vi "Configuration.vi"(10 "Open from\nscan VI":bool, 11 "Measurements":T1(tab)) -> (3 "configured?":bool)   [LabVIEW 2013]
uses:
  InstrControl/Switching/Switching.lvclass
  InstrControl/InstrumentSetup.vi
  general_VIs/globals/QC_MeasurementSetup.vi
  general_VIs/globals/QC_RunInformation.vi
  InstrControl/InstrControl.lvclass
panel:
  in  "Defaults Multimeter":bool
  in  "Multimeter":enum32{"Keithley 2000"}(tab)
  in  "Range Value\n(0.1 - 100)":dbl=100.0 format="%#.2g"
  in  "Range":u16(ring) items=["Auto", "Manual"]
  in  "Function":u16(ring)=3 items=["AC Current", "DC Current", "AC Voltage", "DC Voltage", "2W-Resistance", "4W-Resistance", "Period", "Frequency", "Temperature", "Diode", "Continuity"]
  in  "GPIB Address KE2000":i32=19
  in  "Apply":bool
  in  "Defaults LCR":bool
  in  "LCRs":enum32{"WayneKerr 6440B", "WayneKerr 6425"}(tab)
  in  "AC frequency [Hz]":i32=1000 format="%#.3p"
  in  "RC Configuration":u16(ring) items=["serial", "parallel"]
  in  "AC amplitude [V]":sgl=0.1
  in  "GPIB Address WK6440B":i32=23
  in  "GPIB Address WK6425":i32=17
  in  "AC amplitude [V] WK6425":sgl=0.1 caption="AC amplitude [V]"
  in  "RC Configuration WK6425":u16(ring) caption="RC Configuration" items=["serial", "parallel"]
  in  "AC frequency [Hz] WK6425":i32=1000 caption="AC frequency [Hz]" format="%#.3p"
  in  "VISA address":refnum<visa-resource-name>="COM24" caption="Arduino address"
  out "Programm uploaded?":string="Make sure programme is uploaded to Arduino Uno ->"
  in  "Blank Button":bool
  in  "Matrix address":i32=1
  in  "GPIB address":i32=10
  in  "Mux1 address":i32=4
  in  "Mux2 address":i32=5
  in  "Search Button":bool
  out "DIAGNOSTIC? Response":string
  out "Display Matrix":bool[][](array[boolean])
  in  "No Matrix":bool
  out "X Mapping":string[](array[string])
  out "Y Mapping":string[](array[string])
  in  "Change Preset Parameters":bool
  in  "V_breakdown Limit [V]":dbl=-500.0
  in  "IV Temperature Readout":enum16{"Read Arduino", "Enter manually"}(ring) caption="Temperature Readout"
  in  "IV Ramp down Interval [s]":i32=1 caption="Ramp down Interval [s]"
  in  "IV Ramp down steps [V]":dbl=50.0 caption="Ramp down steps [V]"
  in  "IV Step Interval [s]":i32=10 caption="Step Interval [s]"
  in  "IV Step Size [V]":dbl=10.0 caption="Step Size [V]" format="%.1f"
  in  "IV Final Voltage [V]":dbl=-700.0 caption="Final Voltage [V]" format="%.1f"
  in  "IV Initial Voltage [V]":dbl caption="Initial Voltage [V]" format="%.1f"
  in  "IV Voltage Supply":string(combo)="Keithley 2410"
  in  "Save IV defaults":bool
  in  "V_depletion Limit [V]":dbl=-300.0
  in  "CV LCR Meter":string(combo)="WayneKerr 6440B"
  in  "CV Temperature Readout":enum16{"Read Arduino", "Enter manually"}(ring) caption="Temperature Readout"
  in  "Save CV defaults":bool
  in  "CV Voltage Supply":string(combo)="Keithley 2410"
  in  "CV Initial Voltage [V]":dbl caption="Initial Voltage [V]" format="%.1f"
  in  "CV Final Voltage [V]":dbl=-700.0 caption="Final Voltage [V]" format="%.1f"
  in  "CV Step Size [V]":dbl=10.0 caption="Step Size [V]" format="%.1f"
  in  "CV Step Interval [s]":i32=5 caption="Step Interval [s]"
  in  "CV Ramp down steps [V]":dbl=10.0 caption="Ramp down steps [V]"
  in  "CV Ramp down Interval [s]":i32=1 caption="Ramp down Interval [s]"
  in  "Maximum current fluctuation [%]":dbl=2.0
  in  "Save Stability defaults":bool
  in  "Stability Voltage Supply":string(combo)="Keithley 487"
  in  "Fraction of good strips [%]":dbl=98.0
  in  "Bias Supply":string(combo)="Keithley 487"
  in  "SMU":string(combo)="Keithley 2410"
  in  "C_is Limit [pF/cm]":dbl=1.0
  in  "Save Cis defaults":bool
  in  "Cis Voltage Supply":string(combo)="Keithley 2410"
  in  "Cis Temperature Readout":enum16{"Read Arduino", "Enter manually"}(ring) caption="Temperature Readout"
  in  "Cis LCR Meter":string(combo)="WayneKerr 6440B"
  in  "Cis Ramp down Interval [s]":i32=1 caption="Ramp down Interval [s]"
  in  "Cis Ramp down steps [V]":dbl=50.0 caption="Ramp down steps [V]"
  in  "Cis Step Interval [s]":i32=10 caption="Step Interval [s]"
  in  "Cis Step Size [V]":dbl=10.0 caption="Step Size [V]" format="%.1f"
  in  "Cis Final Voltage [V]":dbl=-700.0 caption="Final Voltage [V]" format="%.1f"
  in  "Cis Initial Voltage [V]":dbl caption="Initial Voltage [V]" format="%.1f"
  in  "Ris Voltmeter":string(combo)="Keithley 2000"
  in  "Ris SMU":string(combo)="Keithley 6517"
  in  "Ris Bias Supply":string(combo)="Keithley 487"
  in  "Ris Temperature Readout":enum16{"Read Arduino", "Enter manually"}(ring) caption="Temperature Readout"
  in  "Save Ris defaults":bool
  in  "Ris Initial Voltage [V]":dbl caption="Initial Voltage [V]" format="%.1f"
  in  "Ris Final Voltage [V]":dbl=-700.0 caption="Final Voltage [V]" format="%.1f"
  in  "Ris Step Size [V]":dbl=10.0 caption="Step Size [V]" format="%.1f"
  in  "Ris Step Interval [s]":i32=10 caption="Step Interval [s]"
  in  "Ris Ramp down steps [V]":dbl=50.0 caption="Ramp down steps [V]"
  in  "Ris Ramp down Interval [s]":i32=1 caption="Ramp down Interval [s]"
  in  "R_is Limit [MOhm]":dbl=100.0
  in  "Supplies":T2(tab)
  in  "Current Limit [µA]":sgl=100.0
  in  "GPIB Address KE2410":i32=24
  in  "GPIB Address KE487":i32=22
  in  "Compliance":u16(ring) items=["20µA", "2mA"]
  in  "Range:":u16(ring) items=["Autorange", "2nA", "20nA", "200nA", "2 microAmp", "20 microAmp", "200 microAmp", "2 milliAmp"]
  in  "Current Limit":u16(ring)=1 items=["OFF", "ON"]
  in  "GPIB Address KE6517":i32=27
  in  "current compliance \nlevel [mA]":dbl=0.0001 format="%.4f"
  in  "compliance/\nmeasurement range (auto:0)":u16(ring)=6 items=["auto / auto", "1 nA / 1.1 V", "10 nA / 11 V", "100 nA / 110 V", "0.001 mA / 110 V", "0.01 mA / 110 V", "0.1 mA / 110 V", "1 mA / 110 V", "10 mA / 110 V", "100 mA / 110 V"]
  in  "GPIB Address KE236":i32=16
  in  "Defaults Supply":bool
  in  "OK Button":bool
  out "X Mapping CB Standard":string[](array[string])
  # "Measurement Configuration"
  # "MUX / Matrix Setup"
  # "Does not apply\nto striptest"
  # "Arduino Configuration"
  # "Multimeter Configuration"
  # "Supply Configuration"
  # "LCR Configuration"
  # "Only for\ninitialisation"
  # "Only for\ninitialisation"
  # "Does not do \nanything yet!"
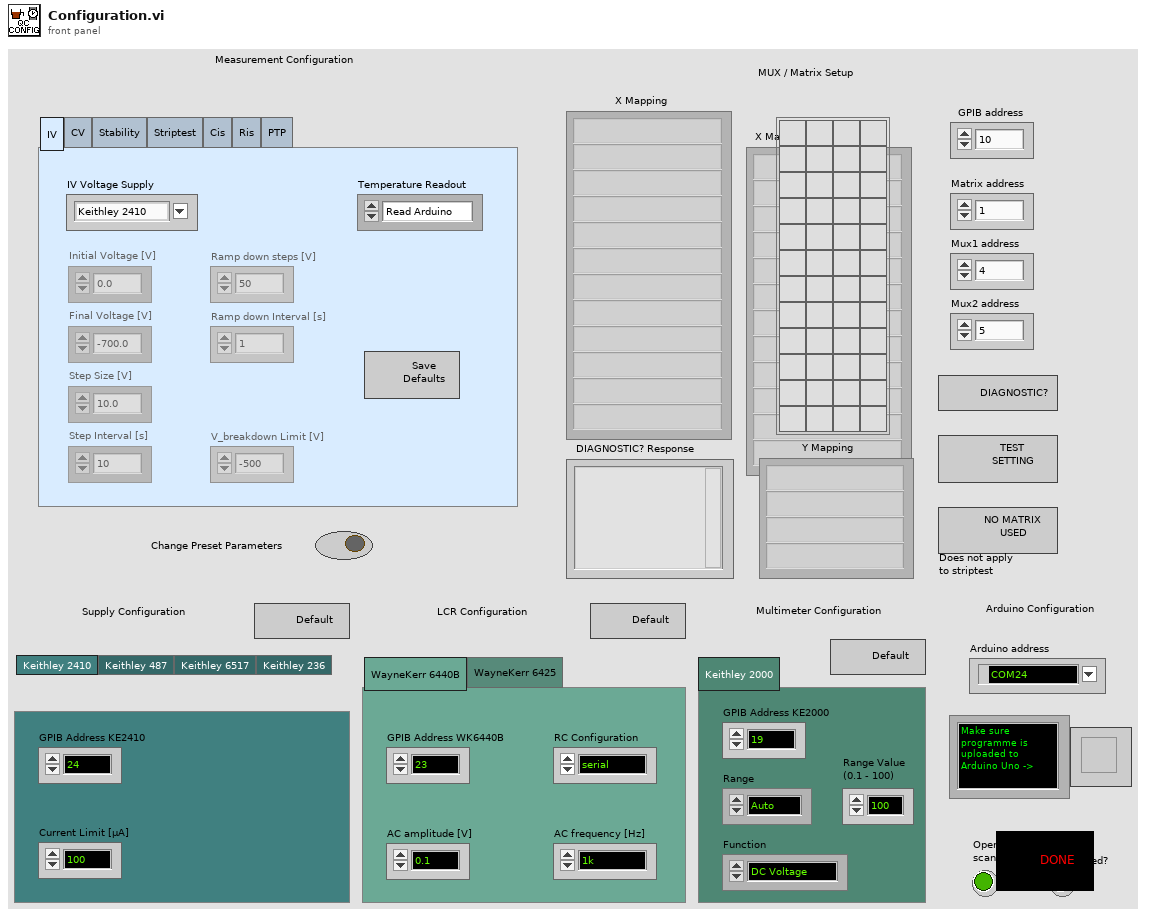
[diagram p1: front panel]
types:
  T1 = enum32{"IV", "CV", "Stability", "Striptest", "Cis", "Ris", "PTP"}
  T2 = enum32{"Keithley 2410", "Keithley 487", "Keithley 6517", "Keithley 236"}
  T3 = enum16{"Reset", "Ground", "Striptest SMU", "Striptest LCR", "IV", "CV", "Interstrip Cap", "Interstrip Res"}
  T4 = cluster{"GPIB address":string, "Matrix address":string, "Mux1 address":string, "Mux2 address":string, "Matrix used?":bool, "Switching":refnum<class "Switching.lvclass">, "Matrix X Channels":cluster{"Bias Supply / SMU LO":i32, "Bias Supply / SMU HI":i32, "CV Box LO":i32, "CV Box HI":i32, "CV Box LO IN":i32, "CV Box HI IN":i32, "Volt meter LO":i32, "Volt meter HI":i32, "Mux1 C1":i32, "Mux1 C2":i32, "Mux2 C1":i32, "Mux2 C2":i32}}
  T5 = cluster{"Supply":refnum<class "SupplyControl.lvclass">, "LCR":refnum<class "LCRControl.lvclass">, "Initial Voltage [V]":dbl, "Final Voltage [V]":dbl, "Step Size [V]":dbl, "Step Interval [s]":i32, "Number Of Steps":u32, "AC frequency [Hz]":i32, "RC Configuration":u16, "AC amplitude [V]":dbl, "Ramp down steps [V]":dbl, "Ramp down Interval [s]":i32, "Set Current Limit?":bool, "Current Limit [µA]":dbl, "Temperature Readout":enum16{"Read Arduino", "Enter manually"}, "Arduino":refnum<class "ArduinoControl.lvclass">, "Supply Name":string, "LCR Name":string, "C_is Limit [pF/cm]":dbl}
  T6 = cluster{"Supply":refnum<class "SupplyControl.lvclass">, "LCR":refnum<class "LCRControl.lvclass">, "Initial Voltage [V]":dbl, "Final Voltage [V]":dbl, "Step Size [V]":dbl, "Step Interval [s]":i32, "Number Of Steps":u32, "AC frequency [Hz]":i32, "RC Configuration":u16, "AC amplitude [V]":dbl, "Ramp down steps [V]":dbl, "Ramp down Interval [s]":i32, "Set Current Limit?":bool, "Current Limit [µA]":dbl, "Temperature Readout":enum16{"Read Arduino", "Enter manually"}, "Arduino":refnum<class "ArduinoControl.lvclass">, "Supply Name":string, "LCR Name":string, "V_depletion Limit [V]":dbl}
  T7 = cluster{"Bias Supply":refnum<class "SupplyControl.lvclass">, "SMU":refnum<class "SupplyControl.lvclass">, "Multimeter":refnum<class "MultimeterControl.lvclass">, "Initial Voltage [V]":dbl, "Final Voltage [V]":dbl, "Step Size [V]":dbl, "Step Interval [s]":i32, "Number Of Steps":u32, "Ramp down steps [V]":dbl, "Ramp down Interval [s]":i32, "Set Current Limit?":bool, "Current Limit [µA]":dbl, "Temperature Readout":enum16{"Read Arduino", "Enter manually"}, "Arduino":refnum<class "ArduinoControl.lvclass">, "Supply Name":string, "SMU Name":string, "Voltmeter Name":string, "R_is Limit [MOhm]":dbl}
  T8 = cluster{"Supply":refnum<class "SupplyControl.lvclass">, "Initial Voltage [V]":dbl, "Final Voltage [V]":dbl, "Step Size [V]":dbl, "Step Interval [s]":i32, "Number Of Steps":u32, "Ramp down steps [V]":dbl, "Ramp down Interval [s]":i32, "Set Current Limit?":bool, "Current Limit [µA]":dbl, "Temperature Readout":enum16{"Read Arduino", "Enter manually"}, "Arduino":refnum<class "ArduinoControl.lvclass">, "Supply Name":string, "V_breakdown Limit [V]":dbl}
  T9 = cluster{"KE 487":string, "KE 6517":string, "WK 6425":string, "KE 236":string, "HP 4263B":string, "KE 2000":string, "KE 2410":string, "WK 6440B":string, "Matrix":string}
  T10 = cluster{"VISA address":refnum<visa-resource-name>, "T sensor":enum16{"SHT", "DS"}, "Arduino":refnum<class "ArduinoControl.lvclass">}
  T11 = cluster{"Range":u16, "Range Value":dbl, "Function":u16, "GPIB Address":string}
  T12 = cluster{"Sensor Serial No.:":string, "Wafer Serial No.:":string, "Batch:":string, "Manufacturer:":string, "Device Category:":string, "Database Serial No.:":string, "Initiated:":string, "Test":string, "Instruments used:":string, "Probeplan used:":string, "End of Run comment:":string, "User:":string}
  T13 = cluster{"RC Configuration":u16, "AC amplitude [V]":dbl, "AC frequency [Hz]":i32, "GPIB Address":string}
  T14 = cluster{"Current Limit":sgl, "GPIB Address":string}
  T15 = cluster{"Compliance":u16, "Range:":u16, "GPIB Address":string}
  T16 = cluster{"Current Limit":u16, "GPIB Address":string}
  T17 = cluster{"current \ncompliance level":dbl, "compliance/\nmeasurement range (auto:0)":u16, "GPIB Address":string}
  T18 = enum16{"Left Button", "Center Button", "Right Button", "Window Close"}
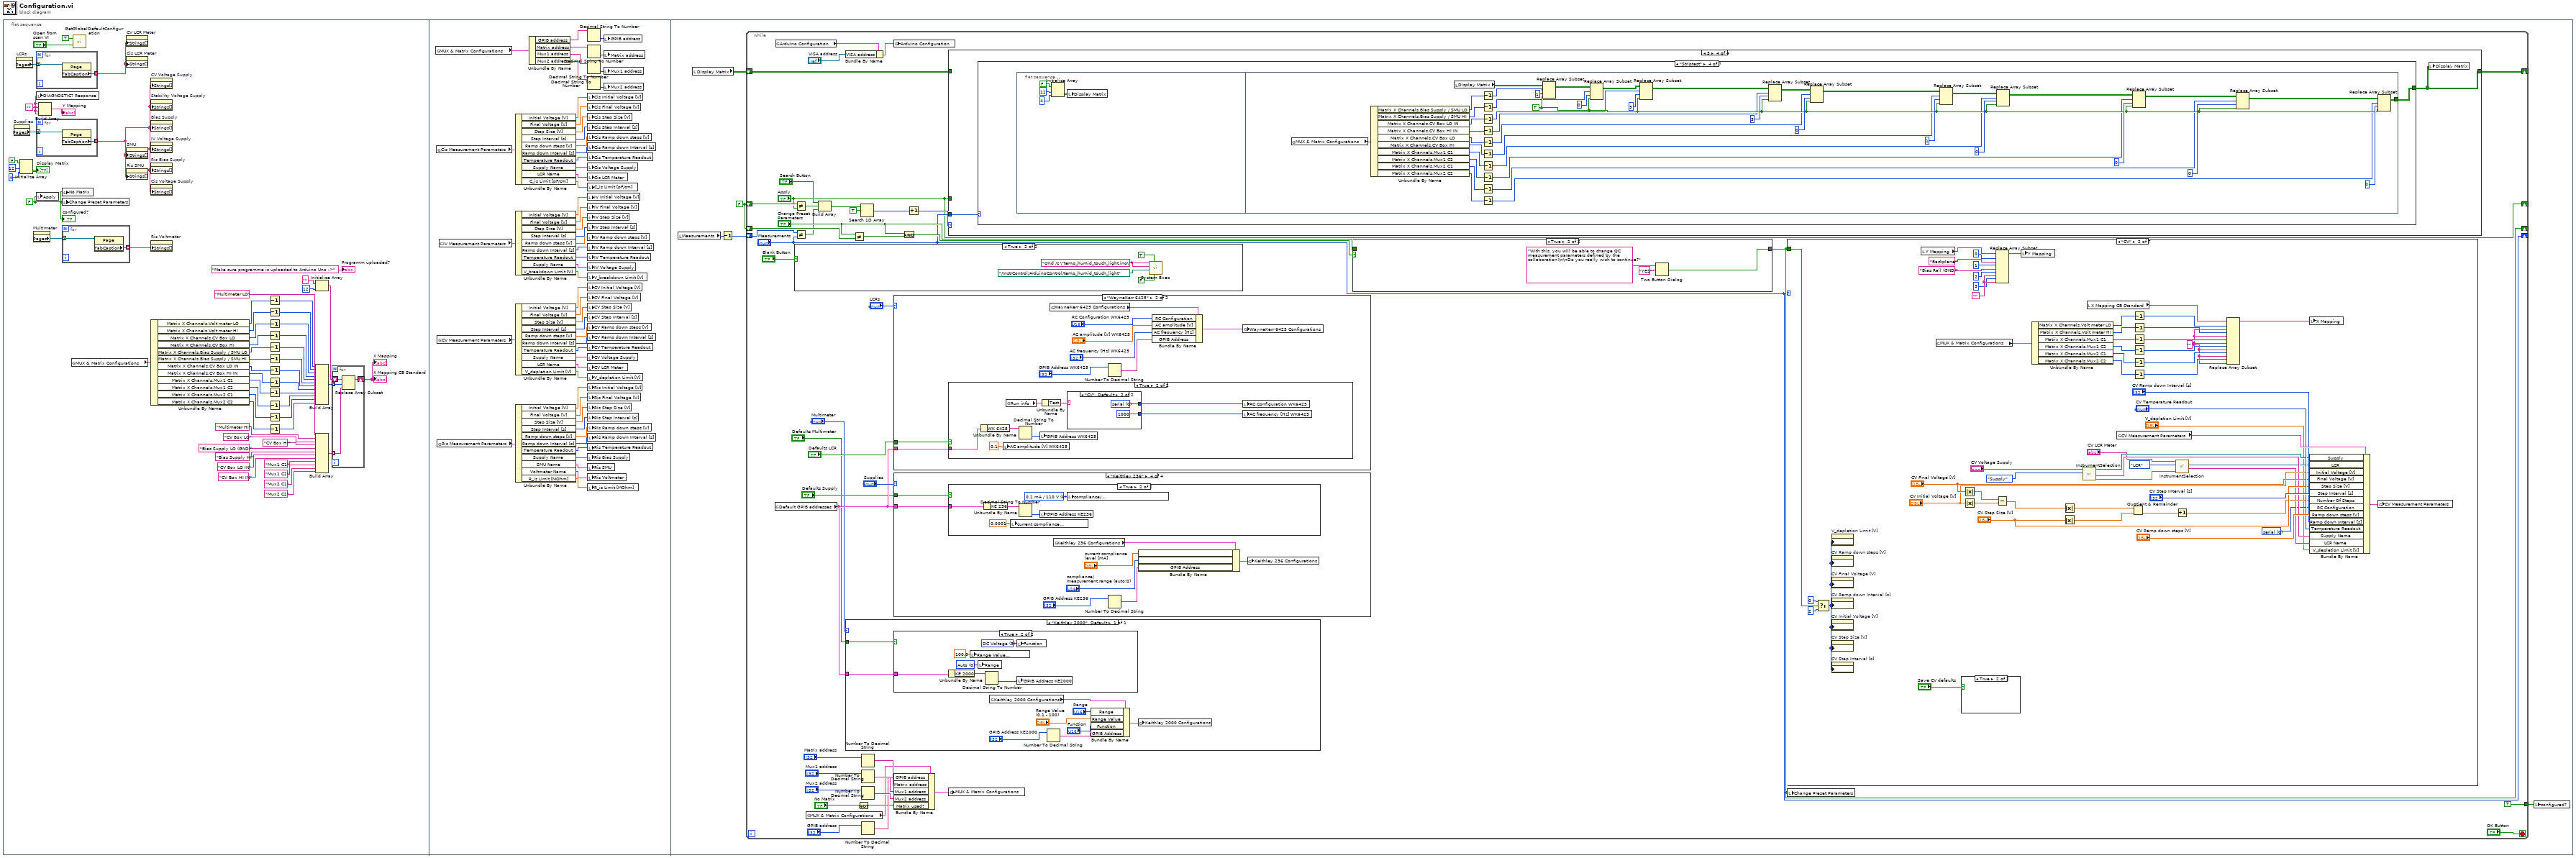
[diagram p0: block diagram]
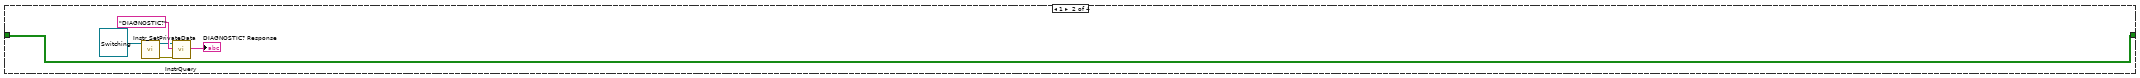
[diagram p3: hidden frame]
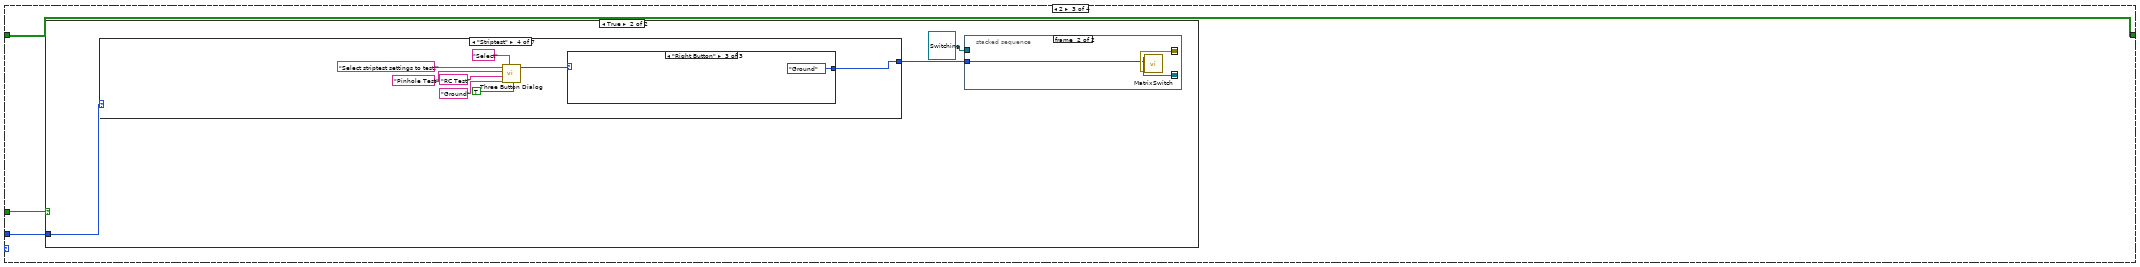
[diagram p4: hidden frame]
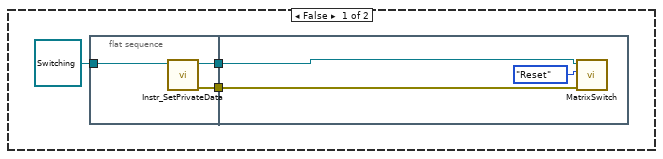
[diagram p5: hidden frame]
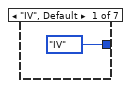
[diagram p6: hidden frame]
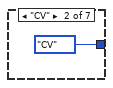
[diagram p7: hidden frame]
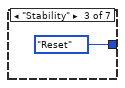
[diagram p8: hidden frame]
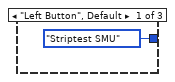
[diagram p9: hidden frame]
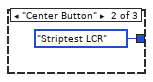
[diagram p10: hidden frame]
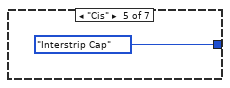
[diagram p11: hidden frame]
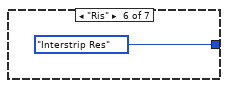
[diagram p12: hidden frame]
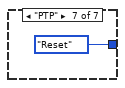
[diagram p13: hidden frame]
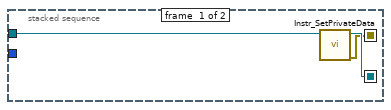
[diagram p14: hidden frame]
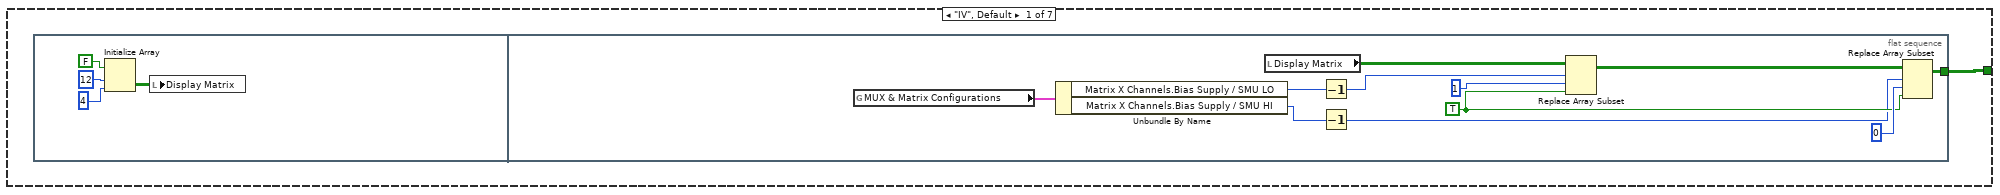
[diagram p15: hidden frame]
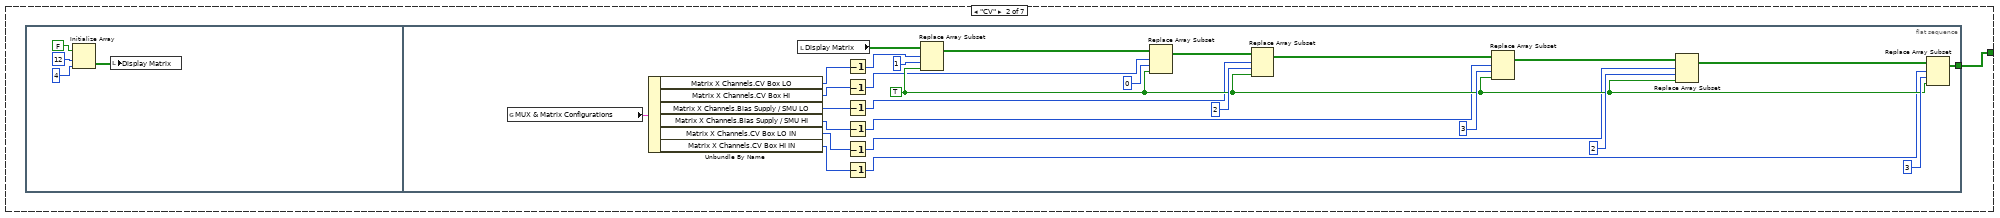
[diagram p16: hidden frame]
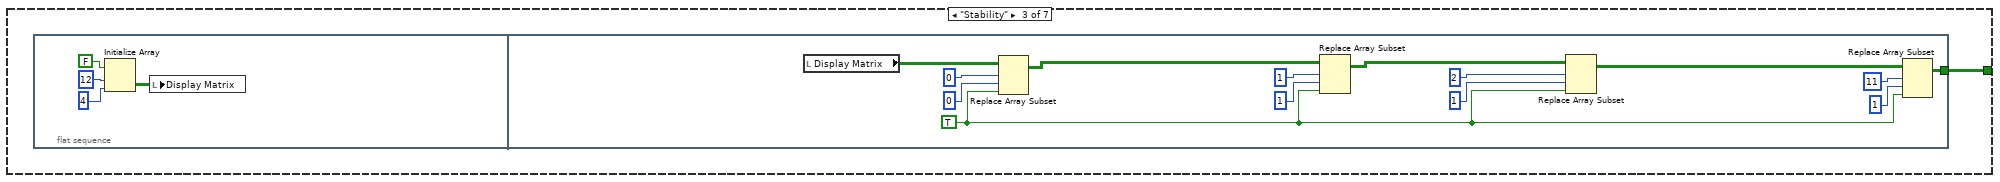
[diagram p17: hidden frame]
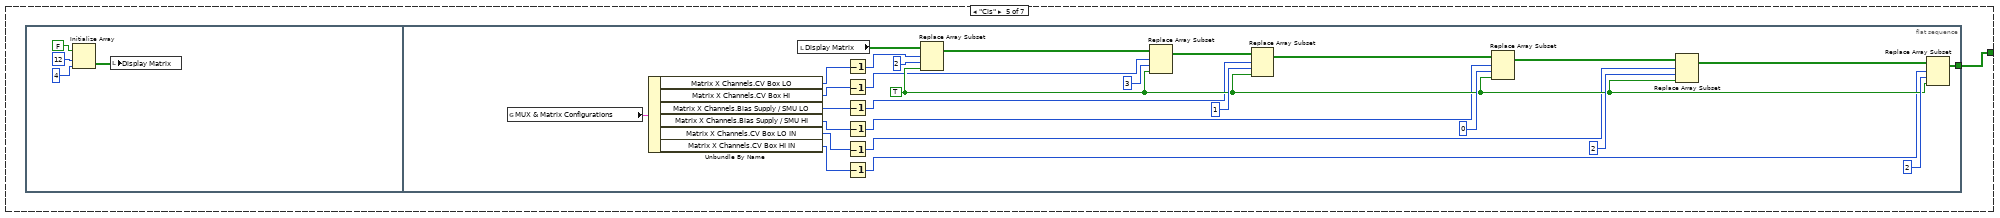
[diagram p18: hidden frame]
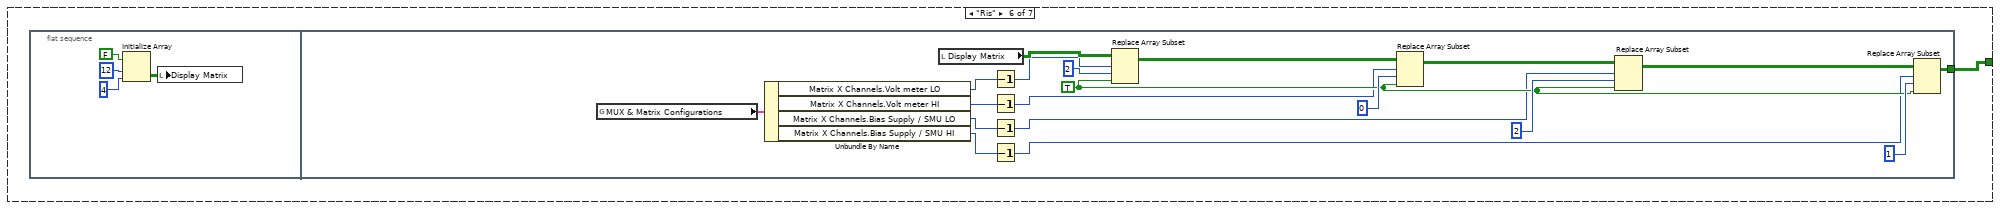
[diagram p19: hidden frame]
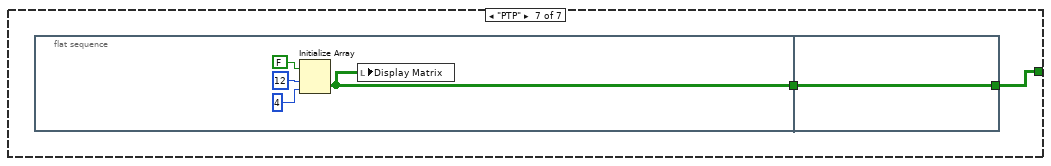
[diagram p20: hidden frame]
diagram:
  n1 = flat-sequence {
    frame #0 {
      w42 = FALSE
      w41 = ""
      n2 = property on="Supplies" class="TabCtl (strict)"() -> ("Pages"=w45:refnum<vi>[])  [unwired: 2 in, 2 out]
      n3 = property on="LCRs" class="TabCtl (strict)"() -> ("Pages"=w44:refnum<vi>[])  [unwired: 2 in, 2 out]
      n4 = Initialize Array(FALSE, 12, 4) -> (→"Display Matrix":bool[][])
      n5 = property on="Multimeter" class="TabCtl (strict)"() -> ("Pages"=w40:refnum<vi>[])  [unwired: 2 in, 2 out]
      n6 = for {
        tunnel: w44 -> [w67] mode=indexing
        tunnel: [w66] -> w43 mode=indexing
        n7 = property class="Page"(reference=w67) -> ("TabCaption"=w66:string)  [unwired: 1 in, 2 out]
      }
      n8 = local write "DIAGNOSTIC? Response"(w41) -> ()
      n9 = for {
        tunnel: w45 -> [w69] mode=indexing
        tunnel: [w68] -> w38 mode=indexing
        n10 = property class="Page"(reference=w69) -> ("TabCaption"=w68:string)  [unwired: 1 in, 2 out]
      }
      n11 = local write "Apply"(w42) -> ()
      n12 = Build Array(w41, w41, w41, w41) -> (→"Y Mapping":string[])
      n13 = local write "No Matrix"(w42) -> ()
      n14 = local write "Change Preset Parameters"(w42) -> ()
      n15 = for {
        tunnel: w40 -> [w65] mode=indexing
        tunnel: [w64] -> w39 mode=indexing
        n16 = property class="Page"(reference=w65) -> ("TabCaption"=w64:string)  [unwired: 1 in, 2 out]
      }
      n17 = global read "InstrumentSetup.vi" "MUX & Matrix Configurations"() -> (w31:T4)
      n18 = call "GetGlobalDefaultConfiguration.vi"("DO NOT override instruments"="Open from\nscan VI", "Read defaults?"=TRUE) -> ()  [unwired: 1 in, 1 out]
      n19 = property on="CV LCR Meter" class="CmbBox"("Strings[]"=w43) -> ()  [unwired: 2 in, 2 out]
      n20 = property on="Cis LCR Meter" class="CmbBox"("Strings[]"=w43) -> ()  [unwired: 2 in, 2 out]
      n21 = property on="SMU" class="CmbBox"("Strings[]"=w38) -> ()  [unwired: 2 in, 2 out]
      n22 = property on="Ris SMU" class="CmbBox"("Strings[]"=w38) -> ()  [unwired: 2 in, 2 out]
      n23 = property on="CV Voltage Supply" class="CmbBox"("Strings[]"=w38) -> ()  [unwired: 2 in, 2 out]
      n24 = property on="Stability Voltage Supply" class="CmbBox"("Strings[]"=w38) -> ()  [unwired: 2 in, 2 out]
      n25 = property on="Bias Supply" class="CmbBox"("Strings[]"=w38) -> ()  [unwired: 2 in, 2 out]
      n26 = property on="IV Voltage Supply" class="CmbBox"("Strings[]"=w38) -> ()  [unwired: 2 in, 2 out]
      n27 = property on="Ris Bias Supply" class="CmbBox"("Strings[]"=w38) -> ()  [unwired: 2 in, 2 out]
      n28 = property on="Cis Voltage Supply" class="CmbBox"("Strings[]"=w38) -> ()  [unwired: 2 in, 2 out]
      n29 = property on="Ris Voltmeter" class="CmbBox"("Strings[]"=w39) -> ()  [unwired: 2 in, 2 out]
      n30 = Unbundle By Name(w31) -> ("Matrix X Channels.Volt meter LO"=w20:i32, "Matrix X Channels.Volt meter HI"=w18:i32, "Matrix X Channels.CV Box LO"=w30:i32, "Matrix X Channels.CV Box HI"=w25:i32, "Matrix X Channels.Bias Supply / SMU LO"=w26:i32, "Matrix X Channels.Bias Supply / SMU HI"=w27:i32, "Matrix X Channels.CV Box LO IN"=w28:i32, "Matrix X Channels.CV Box HI IN"=w29:i32, "Matrix X Channels.Mux1 C1"=w21:i32, "Matrix X Channels.Mux1 C2"=w22:i32, "Matrix X Channels.Mux2 C1"=w23:i32, "Matrix X Channels.Mux2 C2"=w24:i32)
      n31 = Decrement(x=w20) -> (x-1=w19:i32)
      n32 = Decrement(x=w18) -> (x-1=w17:i32)
      n33 = Decrement(x=w30) -> (x-1=w16:i32)
      n34 = Decrement(x=w25) -> (x-1=w15:i32)
      n35 = Decrement(x=w26) -> (x-1=w14:i32)
      n36 = Decrement(x=w27) -> (x-1=w13:i32)
      n37 = Decrement(x=w28) -> (x-1=w12:i32)
      n38 = Decrement(x=w29) -> (x-1=w11:i32)
      n39 = Decrement(x=w21) -> (x-1=w10:i32)
      n40 = Decrement(x=w22) -> (x-1=w9:i32)
      n41 = Decrement(x=w23) -> (x-1=w8:i32)
      n42 = Decrement(x=w24) -> (x-1=w7:i32)
      n43 = Initialize Array("", 12) -> (w2:string[])
      n44 = Build Array(w19, w17, w16, w15, w14, w13, w12, w11, w10, w9, w8, w7) -> (w6:i32[])
      n45 = Build Array("Multimeter LO" ("Input Element"), "Multimeter HI" ("Input Element"), "CV Box LO" ("Input Element"), "CV Box HI" ("Input Element"), "Bias Supply LO (GND)" ("Input Element"), "Bias Supply HI" ("Input Element"), "CV Box LO IN" ("Input Element"), "CV Box HI IN" ("Input Element"), "Mux1 C1" ("String"), "Mux1 C2" ("String"), "Mux2 C1" ("String"), "Mux2 C2" ("String")) -> (w5:string[])
      n46 = for {
        tunnel: w6 -> [w61] mode=indexing
        tunnel: w5 -> [w62] mode=indexing
        shift-right: [w60] -> w1
        shift-left: w2 -> [w63]
        n47 = Replace Array Subset(array=w63, new element=w62, index=w61) -> (w60:string[])
      }
      "X Mapping" <- w1
      "X Mapping CB Standard" <- w1
      "configured?" <- w42
      "Programm uploaded?" <- "Make sure programme is uploaded to Arduino Uno ->"
    }
    frame #1 {
      n48 = global read "InstrumentSetup.vi" "MUX & Matrix Configurations"() -> (w112:T4)
      n49 = global read "QC_MeasurementSetup.vi" "Cis Measurement Parameters"() -> (w93:T5)
      n50 = global read "QC_MeasurementSetup.vi" "CV Measurement Parameters"() -> (w82:T6)
      n51 = global read "QC_MeasurementSetup.vi" "Ris Measurement Parameters"() -> (w81:T7)
      n52 = global read "QC_MeasurementSetup.vi" "IV Measurement Parameters"() -> (w113:T8)
      n53 = Unbundle By Name(w93) -> ("Initial Voltage [V]"=w94:dbl, "Final Voltage [V]"=w95:dbl, "Step Size [V]"=w96:dbl, "Step Interval [s]"=w98:i32, "Ramp down steps [V]"=w97:dbl, "Ramp down Interval [s]"=w99:i32, "Temperature Readout"=w100:enum16{"Read Arduino", "Enter manually"}, "Supply Name"=w101:string, "LCR Name"=w102:string, "C_is Limit [pF/cm]"=w103:dbl)
      n54 = Unbundle By Name(w113) -> ("Initial Voltage [V]"=w114:dbl, "Final Voltage [V]"=w119:dbl, "Step Size [V]"=w120:dbl, "Step Interval [s]"=w116:i32, "Ramp down steps [V]"=w115:dbl, "Ramp down Interval [s]"=w122:i32, "Temperature Readout"=w117:enum16{"Read Arduino", "Enter manually"}, "Supply Name"=w118:string, "V_breakdown Limit [V]"=w121:dbl)
      n55 = Unbundle By Name(w82) -> ("Initial Voltage [V]"=w85:dbl, "Final Voltage [V]"=w86:dbl, "Step Size [V]"=w87:dbl, "Step Interval [s]"=w84:i32, "Ramp down steps [V]"=w88:dbl, "Ramp down Interval [s]"=w92:i32, "Temperature Readout"=w91:enum16{"Read Arduino", "Enter manually"}, "Supply Name"=w89:string, "LCR Name"=w90:string, "V_depletion Limit [V]"=w83:dbl)
      n56 = Unbundle By Name(w81) -> ("Initial Voltage [V]"=w80:dbl, "Final Voltage [V]"=w79:dbl, "Step Size [V]"=w73:dbl, "Step Interval [s]"=w72:i32, "Ramp down steps [V]"=w76:dbl, "Ramp down Interval [s]"=w78:i32, "Temperature Readout"=w71:enum16{"Read Arduino", "Enter manually"}, "Supply Name"=w77:string, "SMU Name"=w75:string, "Voltmeter Name"=w74:string, "R_is Limit [MOhm]"=w70:dbl)
      n57 = Unbundle By Name(w112) -> ("GPIB address"=w111:string, "Matrix address"=w109:string, "Mux1 address"=w108:string, "Mux2 address"=w104:string)
      n58 = Decimal String To Number(string=w111) -> (number=w110:i32)  [unwired: 2 in, 1 out]
      n59 = Decimal String To Number(string=w109) -> (number=w106:i32)  [unwired: 2 in, 1 out]
      n60 = Decimal String To Number(string=w108) -> (number=w105:i32)  [unwired: 2 in, 1 out]
      n61 = Decimal String To Number(string=w104) -> (number=w107:i32)  [unwired: 2 in, 1 out]
      n62 = local write "Cis Initial Voltage [V]"(w94) -> ()
      n63 = local write "Cis Final Voltage [V]"(w95) -> ()
      n64 = local write "Cis Step Size [V]"(w96) -> ()
      n65 = local write "Cis Step Interval [s]"(w98) -> ()
      n66 = local write "Cis Ramp down steps [V]"(w97) -> ()
      n67 = local write "Cis Ramp down Interval [s]"(w99) -> ()
      n68 = local write "Cis Temperature Readout"(w100) -> ()
      n69 = local write "Cis Voltage Supply"(w101) -> ()
      n70 = local write "Cis LCR Meter"(w102) -> ()
      n71 = local write "C_is Limit [pF/cm]"(w103) -> ()
      n72 = local write "IV Initial Voltage [V]"(w114) -> ()
      n73 = local write "IV Final Voltage [V]"(w119) -> ()
      n74 = local write "IV Step Size [V]"(w120) -> ()
      n75 = local write "IV Step Interval [s]"(w116) -> ()
      n76 = local write "IV Ramp down steps [V]"(w115) -> ()
      n77 = local write "IV Ramp down Interval [s]"(w122) -> ()
      n78 = local write "IV Temperature Readout"(w117) -> ()
      n79 = local write "IV Voltage Supply"(w118) -> ()
      n80 = local write "V_breakdown Limit [V]"(w121) -> ()
      n81 = local write "CV Initial Voltage [V]"(w85) -> ()
      n82 = local write "CV Final Voltage [V]"(w86) -> ()
      n83 = local write "CV Step Size [V]"(w87) -> ()
      n84 = local write "CV Step Interval [s]"(w84) -> ()
      n85 = local write "CV Ramp down steps [V]"(w88) -> ()
      n86 = local write "CV Ramp down Interval [s]"(w92) -> ()
      n87 = local write "CV Temperature Readout"(w91) -> ()
      n88 = local write "CV Voltage Supply"(w89) -> ()
      n89 = local write "CV LCR Meter"(w90) -> ()
      n90 = local write "V_depletion Limit [V]"(w83) -> ()
      n91 = local write "Ris Initial Voltage [V]"(w80) -> ()
      n92 = local write "Ris Final Voltage [V]"(w79) -> ()
      n93 = local write "Ris Step Size [V]"(w73) -> ()
      n94 = local write "Ris Step Interval [s]"(w72) -> ()
      n95 = local write "Ris Ramp down steps [V]"(w76) -> ()
      n96 = local write "Ris Ramp down Interval [s]"(w78) -> ()
      n97 = local write "Ris Temperature Readout"(w71) -> ()
      n98 = local write "Ris Bias Supply"(w77) -> ()
      n99 = local write "Ris SMU"(w75) -> ()
      n100 = local write "Ris Voltmeter"(w74) -> ()
      n101 = local write "R_is Limit [MOhm]"(w70) -> ()
      n102 = local write "GPIB address"(w110) -> ()
      n103 = local write "Matrix address"(w106) -> ()
      n104 = local write "Mux1 address"(w105) -> ()
      n105 = local write "Mux2 address"(w107) -> ()
    }
    frame #2 {
      w124 = FALSE
      n106 = local read "Measurements"() -> (w126:T1)
      n107 = local read "Display Matrix"() -> (w123:bool[][])
      n108 = Decrement(x=w126) -> (x-1=w125:T1)
      n109 = while {
        shift-right: [w164] -> _
        shift-left: w124 -> [w167]
        shift-right: ["Measurements"] -> _
        shift-left: w125 -> [w151]
        shift-right: [w129] -> _
        shift-left: w123 -> [w128]
        tunnel: [TRUE] -> w127
        shift-right: ["Apply"] -> _
        shift-left: w124 -> [w145]
        stop <- "OK Button" stop-if-true
        n110 = global read "InstrumentSetup.vi" "Default GPIB addresses"() -> (w143:T9)
        n111 = global read "InstrumentSetup.vi" "Arduino Configuration"() -> (w149:T10)
        n112 = Not Equal?(x=w145, y="Apply") -> (x != y?=w134:bool)
        n113 = Not Equal?(x=w151, y="Measurements") -> (x != y?=w130:bool)
        n114 = case shown="True" "Blank Button" {
          frame False {
          }
          frame True {
            w454 = "cmd /c \"temp_humid_touch_light.ino\""
            n115 = call <vilib>:"System Exec.vi"("run minimized? (F)"=FALSE, "wait until completion? (T)"=TRUE, "working directory"=path "../InstrControl/ArduinoControl/temp_humid_touch_light", "standard input"=w454, "command line"=w454) -> ()  [unwired: 3 in, 4 out]
          }
        }
        n116 = global read "InstrumentSetup.vi" "MUX & Matrix Configurations"() -> (w154:T4)
        n117 = Build Array("Search Button", w134, w130) -> (w136:bool[])
        n118 = Bundle By Name(cluster=w149, "VISA address"="VISA address") -> (w150:T10)
        n119 = case shown="\"Keithley 2000\", Default" "Multimeter" {
          tunnel: "Defaults Multimeter" -> [w404]
          tunnel: w143 -> [w403]
          frame "Keithley 2000", Default {
            n120 = case shown="True" w404 {
              tunnel: w403 -> [_ w410]
              frame False {
              }
              frame True {
                w406 = u16 0 items=["Auto", "Manual"] ("Range")
                w407 = u16 3 items=["AC Current", "DC Current", "AC Voltage", "DC Voltage", "2W-Resistance", "4W-Resistance", "Period", "Frequency", "Temperature", "Diode", "Continuity"] ("Function")
                n121 = Unbundle By Name(w410) -> ("KE 2000"=w409:string)
                n122 = local write "Range Value\n(0.1 - 100)"(100.0 ("Range Value\n(0.1 - 100)")) -> ()
                n123 = local write "Range"(w406) -> ()
                n124 = Decimal String To Number(string=w409) -> (number=w408:i32)  [unwired: 2 in, 1 out]
                n125 = local write "Function"(w407) -> ()
                n126 = local write "GPIB Address KE2000"(w408) -> ()
              }
            }
            n127 = global read "InstrumentSetup.vi" "Keithley 2000 Configurations"() -> (w402:T11)
            n128 = Number To Decimal String(number="GPIB Address KE2000") -> (decimal integer string=w396:string)  [unwired: 1 in]
            n129 = Bundle By Name(cluster=w402, "Range"="Range", "Range Value"="Range Value\n(0.1 - 100)", "Function"="Function", "GPIB Address"=w396) -> (w401:T11)
            n130 = global write "InstrumentSetup.vi" "Keithley 2000 Configurations"(w401) -> ()
          }
        }
        n131 = Not Equal?(x="Change Preset Parameters", y=w167) -> (x != y?=w166:bool)
        n132 = Not(x="No Matrix") -> (.not. x?=w146:bool)
        n133 = Search 1D Array(1D array=w136, element=TRUE) -> (index of element=w138:i32)  [unwired: 1 in]
        n134 = Number To Decimal String(number="Matrix address") -> (decimal integer string=w162:string)  [unwired: 1 in]
        n135 = Number To Decimal String(number="Mux1 address") -> (decimal integer string=w160:string)  [unwired: 1 in]
        n136 = Number To Decimal String(number="Mux2 address") -> (decimal integer string=w161:string)  [unwired: 1 in]
        n137 = Number To Decimal String(number="GPIB address") -> (decimal integer string=w156:string)  [unwired: 1 in]
        n138 = global write "InstrumentSetup.vi" "Arduino Configuration"(w150) -> ()
        n139 = case shown="\"WayneKerr 6425\"" "LCRs" {
          tunnel: "Defaults LCR" -> [w414 w432]
          tunnel: w143 -> [w413 w433]
          frame "WayneKerr 6440B", Default {
            n140 = case shown="True" w414 {
              tunnel: w413 -> [_ w427]
              frame False {
              }
              frame True {
                n141 = Unbundle By Name(w427) -> ("WK 6440B"=w426:string)
                n142 = local write "AC amplitude [V]"(0.1) -> ()
                n143 = global read "QC_RunInformation.vi" "Run info"() -> (w421:T12)
                n144 = Decimal String To Number(string=w426) -> (number=w425:i32)  [unwired: 2 in, 1 out]
                n145 = local write "GPIB Address WK6440B"(w425) -> ()
                n146 = Unbundle By Name(w421) -> ("Test"=w420:string)
                n147 = case shown="\"CV\", Default" w420 {
                  tunnel: [w429 w431] -> w423
                  tunnel: [100000 1000] -> w422
                  frame "Cis" {
                    w429 = u16 1 items=["serial", "parallel"] ("RC Configuration")
                  }
                  frame "CV", Default {
                    w431 = u16 0 items=["serial", "parallel"] ("RC Configuration")
                  }
                }
                n148 = local write "RC Configuration"(w423) -> ()
                n149 = local write "AC frequency [Hz]"(w422) -> ()
              }
            }
            n150 = global read "InstrumentSetup.vi" "WayneKerr 6440B Configurations"() -> (w419:T13)
            n151 = Number To Decimal String(number="GPIB Address WK6440B") -> (decimal integer string=w415:string)  [unwired: 1 in]
            n152 = Bundle By Name(cluster=w419, "RC Configuration"="RC Configuration", "AC amplitude [V]"="AC amplitude [V]", "AC frequency [Hz]"="AC frequency [Hz]", "GPIB Address"=w415) -> (w418:T13)
            n153 = global write "InstrumentSetup.vi" "WayneKerr 6440B Configurations"(w418) -> ()
          }
          frame "WayneKerr 6425" {
            n154 = case shown="True" w432 {
              tunnel: w433 -> [_ w448]
              frame False {
              }
              frame True {
                n155 = Unbundle By Name(w448) -> ("WK 6425"=w447:string)
                n156 = local write "AC amplitude [V] WK6425"(0.1) -> ()
                n157 = global read "QC_RunInformation.vi" "Run info"() -> (w442:T12)
                n158 = Decimal String To Number(string=w447) -> (number=w446:i32)  [unwired: 2 in, 1 out]
                n159 = local write "GPIB Address WK6425"(w446) -> ()
                n160 = Unbundle By Name(w442) -> ("Test"=w441:string)
                n161 = case shown="\"CV\", Default" w441 {
                  tunnel: [w450 w452] -> w444
                  tunnel: [100000 1000] -> w443
                  frame "Cis" {
                    w450 = u16 1 items=["serial", "parallel"] ("RC Configuration")
                  }
                  frame "CV", Default {
                    w452 = u16 0 items=["serial", "parallel"] ("RC Configuration")
                  }
                }
                n162 = local write "RC Configuration WK6425"(w444) -> ()
                n163 = local write "AC frequency [Hz] WK6425"(w443) -> ()
              }
            }
            n164 = global read "InstrumentSetup.vi" "WayneKerr 6425 Configurations"() -> (w436:T13)
            n165 = Number To Decimal String(number="GPIB Address WK6425") -> (decimal integer string=w434:string)  [unwired: 1 in]
            n166 = Bundle By Name(cluster=w436, "RC Configuration"="RC Configuration WK6425", "AC amplitude [V]"="AC amplitude [V] WK6425", "AC frequency [Hz]"="AC frequency [Hz] WK6425", "GPIB Address"=w434) -> (w435:T13)
            n167 = global write "InstrumentSetup.vi" "WayneKerr 6425 Configurations"(w435) -> ()
          }
        }
        n168 = case shown="\"Keithley 236\"" "Supplies" {
          tunnel: "Defaults Supply" -> [w779 w791 w803 w815]
          tunnel: w143 -> [w775 w785 w798 w809]
          frame "Keithley 2410", Default {
            n169 = case shown="True" w779 {
              tunnel: w775 -> [_ w783]
              frame False {
              }
              frame True {
                n170 = Unbundle By Name(w783) -> ("KE 2410"=w782:string)
                n171 = local write "Current Limit [µA]"(100.0) -> ()
                n172 = Decimal String To Number(string=w782) -> (number=w781:i32)  [unwired: 2 in, 1 out]
                n173 = local write "GPIB Address KE2410"(w781) -> ()
              }
            }
            n174 = global read "InstrumentSetup.vi" "Keithley 2410 Configurations"() -> (w778:T14)
            n175 = Divide(x="Current Limit [µA]", y=1000000.0) -> (x/y=w771:dbl)
            n176 = Number To Decimal String(number="GPIB Address KE2410") -> (decimal integer string=w777:string)  [unwired: 1 in]
            n177 = Bundle By Name(cluster=w778, "Current Limit"=w771, "GPIB Address"=w777) -> (w776:T14)
            n178 = global write "InstrumentSetup.vi" "Keithley 2410 Configurations"(w776) -> ()
          }
          frame "Keithley 487" {
            n179 = case shown="True" w791 {
              tunnel: w785 -> [_ w796]
              frame False {
              }
              frame True {
                w792 = u16 0 items=["Autorange", "2nA", "20nA", "200nA", "2 microAmp", "20 microAmp", "200 microAmp", "2 milliAmp"] ("Range:")
                w793 = u16 0 items=["20µA", "2mA"] ("Compliance")
                n180 = Unbundle By Name(w796) -> ("KE 487"=w795:string)
                n181 = local write "Compliance"(w793) -> ()
                n182 = Decimal String To Number(string=w795) -> (number=w794:i32)  [unwired: 2 in, 1 out]
                n183 = local write "GPIB Address KE487"(w794) -> ()
                n184 = local write "Range:"(w792) -> ()
              }
            }
            n185 = global read "InstrumentSetup.vi" "Keithley 487 Configurations"() -> (w790:T15)
            n186 = Number To Decimal String(number="GPIB Address KE487") -> (decimal integer string=w788:string)  [unwired: 1 in]
            n187 = Bundle By Name(cluster=w790, "Compliance"="Compliance", "Range:"="Range:", "GPIB Address"=w788) -> (w789:T15)
            n188 = global write "InstrumentSetup.vi" "Keithley 487 Configurations"(w789) -> ()
          }
          frame "Keithley 6517" {
            n189 = case shown="True" w803 {
              tunnel: w798 -> [_ w807]
              frame False {
              }
              frame True {
                w804 = u16 1 items=["OFF", "ON"] ("Current Limit")
                n190 = Unbundle By Name(w807) -> ("KE 6517"=w805:string)
                n191 = local write "Current Limit"(w804) -> ()
                n192 = Decimal String To Number(string=w805) -> (number=w806:i32)  [unwired: 2 in, 1 out]
                n193 = local write "GPIB Address KE6517"(w806) -> ()
              }
            }
            n194 = global read "InstrumentSetup.vi" "Keithley 6517 Configurations"() -> (w802:T16)
            n195 = Number To Decimal String(number="GPIB Address KE6517") -> (decimal integer string=w799:string)  [unwired: 1 in]
            n196 = Bundle By Name(cluster=w802, "Current Limit"="Current Limit", "GPIB Address"=w799) -> (w801:T16)
            n197 = global write "InstrumentSetup.vi" "Keithley 6517 Configurations"(w801) -> ()
          }
          frame "Keithley 236" {
            n198 = case shown="True" w815 {
              tunnel: w809 -> [_ w820]
              frame False {
              }
              frame True {
                w816 = u16 6 items=["auto / auto", "1 nA / 1.1 V", "10 nA / 11 V", "100 nA / 110 V", "0.001 mA / 110 V", "0.01 mA / 110 V", "0.1 mA / 110 V", "1 mA / 110 V", "10 mA / 110 V", "100 mA / 110 V"] ("compliance/\nmeasurement range (auto:0)")
                n199 = Unbundle By Name(w820) -> ("KE 236"=w819:string)
                n200 = local write "current compliance \nlevel [mA]"(0.0001 ("current \ncompliance level")) -> ()
                n201 = Decimal String To Number(string=w819) -> (number=w818:i32)  [unwired: 2 in, 1 out]
                n202 = local write "GPIB Address KE236"(w818) -> ()
                n203 = local write "compliance/\nmeasurement range (auto:0)"(w816) -> ()
              }
            }
            n204 = global read "InstrumentSetup.vi" "Keithley 236 Configurations"() -> (w810:T17)
            n205 = Number To Decimal String(number="GPIB Address KE236") -> (decimal integer string=w814:string)  [unwired: 1 in]
            n206 = Bundle By Name(cluster=w810, "current \ncompliance level"="current compliance \nlevel [mA]", "compliance/\nmeasurement range (auto:0)"="compliance/\nmeasurement range (auto:0)", "GPIB Address"=w814) -> (w811:T17)
            n207 = global write "InstrumentSetup.vi" "Keithley 236 Configurations"(w811) -> ()
          }
        }
        n208 = Bundle By Name(cluster=w154, "GPIB address"=w156, "Matrix address"=w162, "Mux1 address"=w160, "Mux2 address"=w161, "Matrix used?"=w146) -> (w153:T4)
        n209 = And(x="Change Preset Parameters", y=w166) -> (x .and. y?=w168:bool)
        n210 = Increment(x=w138) -> (x+1=w135:i32)
        n211 = case shown="3" w135 {
          tunnel: "Measurements" -> [_ _ w179 w217]
          tunnel: "Apply" -> [_ _ w180 _]
          tunnel: [w171 w172 w178 w216] -> w129
          tunnel: w128 -> [w171 w172 w178 _]
          frame 0, Default {
          }
          frame 1 {
            n212 = call-dynamic "Instr_SetPrivateData.vi"("Switching in"=refnum<class "Switching.lvclass"> refnum ("Switching.lvclass")) -> ("error out"=w175:errorcluster, "Switching out"=w173:refnum<class "Switching.lvclass">)  [unwired: 9 in]
            n213 = call-dynamic "InstrQuery.vi"("error in (no error)"=w175, "Command string"="DIAGNOSTIC?", "InstControl in"=w173) -> ("Instrument response"=→"DIAGNOSTIC? Response":string)  [unwired: 6 in, 2 out]
          }
          frame 2 {
            n214 = case shown="True" w180 {
              tunnel: w179 -> [_ w191]
              frame False {
                n215 = flat-sequence {
                  tunnel: refnum<class "Switching.lvclass"> refnum ("Switching in") -> [w184]
                  tunnel: [w186] -> w182
                  tunnel: [w185] -> w181
                  tunnel: w182 -> [w189]
                  tunnel: w181 -> [w188]
                  frame #0 {
                    n216 = call-dynamic "Instr_SetPrivateData.vi"("Switching in"=w184) -> ("error out"=w185:errorcluster, "Switching out"=w186:refnum<class "Switching.lvclass">)  [unwired: 9 in]
                  }
                  frame #1 {
                    n217 = call "MatrixSwitch.vi"("error in (no error)"=w188, "Action"=T3."Reset", "Switching in"=w189) -> ()  [unwired: 7 in, 2 out]
                  }
                }
              }
              frame True {
                n218 = case shown="\"Striptest\"" w191 {
                  tunnel: [T3."IV" ("Action") T3."CV" ("Action") T3."Reset" ("Action") w201 T3."Interstrip Cap" ("Action") T3."Interstrip Res" ("Action") T3."Reset" ("Action")] -> w190
                  frame "IV", Default {
                  }
                  frame "CV" {
                  }
                  frame "Stability" {
                  }
                  frame "Striptest" {
                    n219 = call <vilib>:"Three Button Dialog.vi"("Allow user to close window? (TRUE)"=TRUE, "Window Title (\"\")"="Select", "Right Button Text (\"Cancel\")"="Ground", "Center Button Text (\"No\")"="RC Test", "Left Button Text (\"Yes\")"="Pinhole Test", "message"="Select striptest settings to test!") -> ("Which Button?"=w203:T18)  [unwired: 5 in]
                    n220 = case shown="\"Right Button\"" w203 {
                      tunnel: [T3."Striptest SMU" ("Action") T3."Striptest LCR" ("Action") T3."Ground" ("Action")] -> w201
                      frame "Left Button", Default {
                      }
                      frame "Center Button" {
                      }
                      frame "Right Button" {
                      }
                    }
                  }
                  frame "Cis" {
                  }
                  frame "Ris" {
                  }
                  frame "PTP" {
                  }
                }
                n221 = stacked-sequence {
                  seq-local: [w212 _] -> [_ w215]
                  seq-local: [w211 _] -> [_ w214]
                  tunnel: refnum<class "Switching.lvclass"> refnum ("Switching in") -> [w210 _]
                  tunnel: w190 -> [_ w213]
                  frame #0 {
                    n222 = call-dynamic "Instr_SetPrivateData.vi"("Switching in"=w210) -> ("error out"=w211:errorcluster, "Switching out"=w212:refnum<class "Switching.lvclass">)  [unwired: 9 in]
                  }
                  frame #1 {
                    n223 = call "MatrixSwitch.vi"("error in (no error)"=w214, "Action"=w213, "Switching in"=w215) -> ()  [unwired: 7 in, 2 out]
                  }
                }
              }
            }
          }
          frame 3 {
            n224 = case shown="\"Striptest\"" w217 {
              tunnel: [w218 w234 w266 w285 w333 w365 w389] -> w216
              frame "IV", Default {
                n225 = flat-sequence {
                  tunnel: [w228] -> w218
                  frame #0 {
                    n226 = Initialize Array(FALSE, 12, 4) -> (w220:bool[][])
                    n227 = local write "Display Matrix"(w220) -> ()
                  }
                  frame #1 {
                    w230 = TRUE
                    n228 = global read "InstrumentSetup.vi" "MUX & Matrix Configurations"() -> (w227:T4)
                    n229 = Unbundle By Name(w227) -> ("Matrix X Channels.Bias Supply / SMU LO"=w226:i32, "Matrix X Channels.Bias Supply / SMU HI"=w225:i32)
                    n230 = local read "Display Matrix"() -> (w229:bool[][])
                    n231 = Decrement(x=w226) -> (x-1=w223:i32)
                    n232 = Decrement(x=w225) -> (x-1=w224:i32)
                    n233 = Replace Array Subset(array=w229, new element=w230, index (row)=w223, index (col)=1) -> (w231:bool[][])
                    n234 = Replace Array Subset(array=w231, new element=w230, index (row)=w224, index (col)=0) -> (w228:bool[][])
                  }
                }
              }
              frame "CV" {
                n235 = flat-sequence {
                  tunnel: [w252] -> w234
                  frame #0 {
                    n236 = Initialize Array(FALSE, 12, 4) -> (w236:bool[][])
                    n237 = local write "Display Matrix"(w236) -> ()
                  }
                  frame #1 {
                    w254 = TRUE
                    n238 = global read "InstrumentSetup.vi" "MUX & Matrix Configurations"() -> (w251:T4)
                    n239 = Unbundle By Name(w251) -> ("Matrix X Channels.CV Box LO"=w250:i32, "Matrix X Channels.CV Box HI"=w245:i32, "Matrix X Channels.Bias Supply / SMU LO"=w246:i32, "Matrix X Channels.Bias Supply / SMU HI"=w247:i32, "Matrix X Channels.CV Box LO IN"=w248:i32, "Matrix X Channels.CV Box HI IN"=w249:i32)
                    n240 = local read "Display Matrix"() -> (w253:bool[][])
                    n241 = Decrement(x=w250) -> (x-1=w244:i32)
                    n242 = Decrement(x=w245) -> (x-1=w243:i32)
                    n243 = Decrement(x=w246) -> (x-1=w242:i32)
                    n244 = Decrement(x=w247) -> (x-1=w241:i32)
                    n245 = Decrement(x=w248) -> (x-1=w240:i32)
                    n246 = Decrement(x=w249) -> (x-1=w239:i32)
                    n247 = Replace Array Subset(array=w253, new element=w254, index (row)=w244, index (col)=1) -> (w263:bool[][])
                    n248 = Replace Array Subset(array=w263, new element=w254, index (row)=w243, index (col)=0) -> (w262:bool[][])
                    n249 = Replace Array Subset(array=w262, new element=w254, index (row)=w242, index (col)=2 ("Index")) -> (w261:bool[][])
                    n250 = Replace Array Subset(array=w261, new element=w254, index (row)=w241, index (col)=3 ("Index")) -> (w255:bool[][])
                    n251 = Replace Array Subset(array=w255, new element=w254, index (row)=w240, index (col)=2) -> (w256:bool[][])
                    n252 = Replace Array Subset(array=w256, new element=w254, index (row)=w239, index (col)=3) -> (w252:bool[][])
                  }
                }
              }
              frame "Stability" {
                n253 = flat-sequence {
                  tunnel: [w271] -> w266
                  frame #0 {
                    n254 = Initialize Array(FALSE, 12, 4) -> (w268:bool[][])
                    n255 = local write "Display Matrix"(w268) -> ()
                  }
                  frame #1 {
                    w272 = TRUE
                    n256 = local read "Display Matrix"() -> (w284:bool[][])
                    n257 = Replace Array Subset(array=w284, new element=w272, index (row)=0, index (col)=0) -> (w281:bool[][])
                    n258 = Replace Array Subset(array=w281, new element=w272, index (row)=1, index (col)=1) -> (w274:bool[][])
                    n259 = Replace Array Subset(array=w274, new element=w272, index (row)=2, index (col)=1) -> (w273:bool[][])
                    n260 = Replace Array Subset(array=w273, new element=w272, index (row)=11, index (col)=1) -> (w271:bool[][])
                  }
                }
              }
              frame "Striptest" {
                n261 = flat-sequence {
                  tunnel: [w311] -> w285
                  frame #0 {
                    n262 = Initialize Array(FALSE, 12, 4) -> (w287:bool[][])
                    n263 = local write "Display Matrix"(w287) -> ()
                  }
                  frame #1 {
                    w313 = TRUE
                    n264 = global read "InstrumentSetup.vi" "MUX & Matrix Configurations"() -> (w310:T4)
                    n265 = Unbundle By Name(w310) -> ("Matrix X Channels.Bias Supply / SMU LO"=w309:i32, "Matrix X Channels.Bias Supply / SMU HI"=w304:i32, "Matrix X Channels.CV Box LO IN"=w305:i32, "Matrix X Channels.CV Box HI IN"=w306:i32, "Matrix X Channels.CV Box LO"=w307:i32, "Matrix X Channels.CV Box HI"=w308:i32, "Matrix X Channels.Mux1 C1"=w300:i32, "Matrix X Channels.Mux1 C2"=w301:i32, "Matrix X Channels.Mux2 C1"=w302:i32, "Matrix X Channels.Mux2 C2"=w303:i32)
                    n266 = local read "Display Matrix"() -> (w321:bool[][])
                    n267 = Decrement(x=w309) -> (x-1=w299:i32)
                    n268 = Decrement(x=w304) -> (x-1=w298:i32)
                    n269 = Decrement(x=w305) -> (x-1=w297:i32)
                    n270 = Decrement(x=w306) -> (x-1=w296:i32)
                    n271 = Decrement(x=w307) -> (x-1=w295:i32)
                    n272 = Decrement(x=w308) -> (x-1=w294:i32)
                    n273 = Decrement(x=w300) -> (x-1=w293:i32)
                    n274 = Decrement(x=w301) -> (x-1=w292:i32)
                    n275 = Decrement(x=w302) -> (x-1=w291:i32)
                    n276 = Decrement(x=w303) -> (x-1=w290:i32)
                    n277 = Replace Array Subset(array=w321, new element=w313, index (row)=w299, index (col)=1) -> (w330:bool[][])
                    n278 = Replace Array Subset(array=w330, new element=w313, index (row)=w298, index (col)=0) -> (w329:bool[][])
                    n279 = Replace Array Subset(array=w329, new element=w313, index (row)=w297, index (col)=3 ("Index")) -> (w328:bool[][])
                    n280 = Replace Array Subset(array=w328, new element=w313, index (row)=w296, index (col)=3 ("Index")) -> (w322:bool[][])
                    n281 = Replace Array Subset(array=w322, new element=w313, index (row)=w295, index (col)=0) -> (w323:bool[][])
                    n282 = Replace Array Subset(array=w323, new element=w313, index (row)=w294, index (col)=1) -> (w312:bool[][])
                    n283 = Replace Array Subset(array=w312, new element=w313, index (row)=w293, index (col)=0) -> (w316:bool[][])
                    n284 = Replace Array Subset(array=w316, new element=w313, index (row)=w292, index (col)=0) -> (w315:bool[][])
                    n285 = Replace Array Subset(array=w315, new element=w313, index (row)=w291, index (col)=0) -> (w314:bool[][])
                    n286 = Replace Array Subset(array=w314, new element=w313, index (row)=w290, index (col)=0) -> (w311:bool[][])
                  }
                }
              }
              frame "Cis" {
                n287 = flat-sequence {
                  tunnel: [w338] -> w333
                  frame #0 {
                    n288 = Initialize Array(FALSE, 12, 4) -> (w335:bool[][])
                    n289 = local write "Display Matrix"(w335) -> ()
                  }
                  frame #1 {
                    w354 = TRUE
                    n290 = global read "InstrumentSetup.vi" "MUX & Matrix Configurations"() -> (w353:T4)
                    n291 = Unbundle By Name(w353) -> ("Matrix X Channels.CV Box LO"=w352:i32, "Matrix X Channels.CV Box HI"=w347:i32, "Matrix X Channels.Bias Supply / SMU LO"=w348:i32, "Matrix X Channels.Bias Supply / SMU HI"=w349:i32, "Matrix X Channels.CV Box LO IN"=w350:i32, "Matrix X Channels.CV Box HI IN"=w351:i32)
                    n292 = local read "Display Matrix"() -> (w344:bool[][])
                    n293 = Decrement(x=w352) -> (x-1=w346:i32)
                    n294 = Decrement(x=w347) -> (x-1=w345:i32)
                    n295 = Decrement(x=w348) -> (x-1=w342:i32)
                    n296 = Decrement(x=w349) -> (x-1=w341:i32)
                    n297 = Decrement(x=w350) -> (x-1=w340:i32)
                    n298 = Decrement(x=w351) -> (x-1=w339:i32)
                    n299 = Replace Array Subset(array=w344, new element=w354, index (row)=w346, index (col)=2) -> (w355:bool[][])
                    n300 = Replace Array Subset(array=w355, new element=w354, index (row)=w345, index (col)=3) -> (w343:bool[][])
                    n301 = Replace Array Subset(array=w343, new element=w354, index (row)=w342, index (col)=1) -> (w362:bool[][])
                    n302 = Replace Array Subset(array=w362, new element=w354, index (row)=w341, index (col)=0) -> (w361:bool[][])
                    n303 = Replace Array Subset(array=w361, new element=w354, index (row)=w340, index (col)=2 ("Index")) -> (w360:bool[][])
                    n304 = Replace Array Subset(array=w360, new element=w354, index (row)=w339, index (col)=2 ("Index")) -> (w338:bool[][])
                  }
                }
              }
              frame "Ris" {
                n305 = flat-sequence {
                  tunnel: [w379] -> w365
                  frame #0 {
                    n306 = Initialize Array(FALSE, 12, 4) -> (w367:bool[][])
                    n307 = local write "Display Matrix"(w367) -> ()
                  }
                  frame #1 {
                    w380 = TRUE
                    n308 = global read "InstrumentSetup.vi" "MUX & Matrix Configurations"() -> (w378:T4)
                    n309 = Unbundle By Name(w378) -> ("Matrix X Channels.Volt meter LO"=w377:i32, "Matrix X Channels.Volt meter HI"=w374:i32, "Matrix X Channels.Bias Supply / SMU LO"=w375:i32, "Matrix X Channels.Bias Supply / SMU HI"=w376:i32)
                    n310 = local read "Display Matrix"() -> (w388:bool[][])
                    n311 = Decrement(x=w377) -> (x-1=w370:i32)
                    n312 = Decrement(x=w374) -> (x-1=w371:i32)
                    n313 = Decrement(x=w375) -> (x-1=w373:i32)
                    n314 = Decrement(x=w376) -> (x-1=w372:i32)
                    n315 = Replace Array Subset(array=w388, new element=w380, index (row)=w370, index (col)=2) -> (w386:bool[][])
                    n316 = Replace Array Subset(array=w386, new element=w380, index (row)=w371, index (col)=0) -> (w383:bool[][])
                    n317 = Replace Array Subset(array=w383, new element=w380, index (row)=w373, index (col)=2) -> (w381:bool[][])
                    n318 = Replace Array Subset(array=w381, new element=w380, index (row)=w372, index (col)=1) -> (w379:bool[][])
                  }
                }
              }
              frame "PTP" {
                n319 = flat-sequence {
                  tunnel: [w391] -> w390
                  tunnel: w390 -> [w395]
                  tunnel: [w395] -> w389
                  frame #0 {
                    n320 = Initialize Array(FALSE, 12, 4) -> (w391:bool[][])
                    n321 = local write "Display Matrix"(w391) -> ()
                  }
                  frame #1 {
                  }
                }
              }
            }
            n322 = local write "Display Matrix"(w216) -> ()
          }
        }
        n323 = global write "InstrumentSetup.vi" "MUX & Matrix Configurations"(w153) -> ()
        n324 = case shown="True" w168 {
          tunnel: [w457 w458] -> w164
          tunnel: "Change Preset Parameters" -> [w457 _]
          frame False {
          }
          frame True {
            n325 = Two Button Dialog(message="With this, you will be able to change QC measurement parameters defined by the collaboration!\n\nDo you really wish to continue?", 2:"YES") -> (T button?=w458:bool)  [unwired: 1 in]
          }
        }
        n326 = case shown="\"CV\"" "Measurements" {
          tunnel: w164 -> [w498 w554 w592 w629 w687 w727 _]
          frame "IV", Default {
            w462 = "" ("Input Element")
            w493 = ""
            n327 = Select(t=0, s=w498, f=2) -> (s? t:f=w496:i32)
            n328 = property on="V_breakdown Limit [V]" class="DigNum (strict)"("DisabledEnum"=w496) -> ()  [unwired: 2 in, 2 out]
            n329 = property on="IV Ramp down Interval [s]" class="DigNum (strict)"("DisabledEnum"=w496) -> ()  [unwired: 2 in, 2 out]
            n330 = property on="IV Step Size [V]" class="DigNum (strict)"("DisabledEnum"=w496) -> ()  [unwired: 2 in, 2 out]
            n331 = property on="IV Ramp down steps [V]" class="DigNum (strict)"("DisabledEnum"=w496) -> ()  [unwired: 2 in, 2 out]
            n332 = property on="IV Final Voltage [V]" class="DigNum (strict)"("DisabledEnum"=w496) -> ()  [unwired: 2 in, 2 out]
            n333 = property on="IV Initial Voltage [V]" class="DigNum (strict)"("DisabledEnum"=w496) -> ()  [unwired: 2 in, 2 out]
            n334 = property on="IV Step Interval [s]" class="DigNum (strict)"("DisabledEnum"=w496) -> ()  [unwired: 2 in, 2 out]
            n335 = local read "Y Mapping"() -> (w487:string[])
            n336 = global read "InstrumentSetup.vi" "MUX & Matrix Configurations"() -> (w473:T4)
            n337 = case shown="True" "Save IV defaults" {
              frame False {
              }
              frame True {
              }
            }
            n338 = Absolute Value(x="IV Final Voltage [V]") -> (abs(x)=w505:dbl)
            n339 = Absolute Value(x="IV Initial Voltage [V]") -> (abs(x)=w504:dbl)
            n340 = Replace Array Subset(array=w487, new element #1="Backplane" ("String"), index #1=0, new element #2="Bias Rail (GND)" ("String"), index #2=1, new element #3=w493, index #3=2, new element #4=w493, index #4=3) -> (w488:string[])
            n341 = Subtract(x=w505, y=w504) -> (x-y=w503:dbl)
            n342 = local write "Y Mapping"(w488) -> ()
            n343 = Unbundle By Name(w473) -> ("Matrix X Channels.CV Box LO"=w467:i32, "Matrix X Channels.CV Box HI"=w468:i32, "Matrix X Channels.CV Box LO IN"=w469:i32, "Matrix X Channels.CV Box HI IN"=w466:i32, "Matrix X Channels.Volt meter LO"=w471:i32, "Matrix X Channels.Volt meter HI"=w470:i32, "Matrix X Channels.Mux1 C1"=w477:i32, "Matrix X Channels.Mux1 C2"=w478:i32, "Matrix X Channels.Mux2 C1"=w475:i32, "Matrix X Channels.Mux2 C2"=w476:i32)
            n344 = Absolute Value(x="IV Step Size [V]") -> (abs(x)=w508:dbl)
            n345 = Absolute Value(x=w503) -> (abs(x)=w502:dbl)
            n346 = local read "X Mapping CB Standard"() -> (w474:string[])
            n347 = global read "QC_MeasurementSetup.vi" "IV Measurement Parameters"() -> (w516:T8)
            n348 = Quotient & Remainder(x=w502, y=w508) -> (floor(x/y)=w500:dbl)  [unwired: 1 out]
            n349 = Decrement(x=w467) -> (x-1=w461:i32)
            n350 = Decrement(x=w468) -> (x-1=w463:i32)
            n351 = Decrement(x=w469) -> (x-1=w464:i32)
            n352 = Decrement(x=w466) -> (x-1=w465:i32)
            n353 = Decrement(x=w471) -> (x-1=w479:i32)
            n354 = Decrement(x=w470) -> (x-1=w480:i32)
            n355 = Decrement(x=w477) -> (x-1=w481:i32)
            n356 = Decrement(x=w478) -> (x-1=w482:i32)
            n357 = Decrement(x=w475) -> (x-1=w483:i32)
            n358 = Decrement(x=w476) -> (x-1=w484:i32)
            n359 = Increment(x=w500) -> (x+1=w499:dbl)
            n360 = call "InstrumentSelection.vi"("Instrument type"=enum16{"Supply", "LCR", "Multimeter"}."Supply", "Instrument name IN"="IV Voltage Supply") -> ("Instrument name OUT"=w511:string, "Supply"=w512:refnum<class "SupplyControl.lvclass">)  [unwired: 5 in, 3 out]
            n361 = Bundle By Name(cluster=w516, "Supply"=w512, "Initial Voltage [V]"="IV Initial Voltage [V]", "Final Voltage [V]"="IV Final Voltage [V]", "Step Size [V]"="IV Step Size [V]", "Step Interval [s]"="IV Step Interval [s]", "Number Of Steps"=w499, "Ramp down steps [V]"="IV Ramp down steps [V]", "Ramp down Interval [s]"="IV Ramp down Interval [s]", "Temperature Readout"="IV Temperature Readout", "Supply Name"=w511, "V_breakdown Limit [V]"="V_breakdown Limit [V]") -> (w517:T8)
            n362 = Replace Array Subset(array=w474, new element #1=w462, index #1=w461, new element #2=w462, index #2=w463, new element #3=w462, index #3=w464, new element #4=w462, index #4=w465, new element #5=w462, index #5=w479, new element #6=w462, index #6=w480, new element #7=w462, index #7=w481, new element #8=w462, index #8=w482, new element #9=w462, index #9=w483, new element #10=w462, index #10=w484) -> (w472:string[])
            n363 = local write "X Mapping"(w472) -> ()
            n364 = global write "QC_MeasurementSetup.vi" "IV Measurement Parameters"(w517) -> ()
          }
          frame "CV" {
            w529 = "" ("Input Element")
            w544 = ""
            w549 = u16 0 items=["serial", "parallel"] ("RC Configuration")
            n365 = Select(t=0, s=w554, f=2) -> (s? t:f=w547:i32)
            n366 = property on="V_depletion Limit [V]" class="DigNum (strict)"("DisabledEnum"=w547) -> ()  [unwired: 2 in, 2 out]
            n367 = property on="CV Ramp down steps [V]" class="DigNum (strict)"("DisabledEnum"=w547) -> ()  [unwired: 2 in, 2 out]
            n368 = property on="CV Final Voltage [V]" class="DigNum (strict)"("DisabledEnum"=w547) -> ()  [unwired: 2 in, 2 out]
            n369 = property on="CV Ramp down Interval [s]" class="DigNum (strict)"("DisabledEnum"=w547) -> ()  [unwired: 2 in, 2 out]
            n370 = property on="CV Initial Voltage [V]" class="DigNum (strict)"("DisabledEnum"=w547) -> ()  [unwired: 2 in, 2 out]
            n371 = property on="CV Step Size [V]" class="DigNum (strict)"("DisabledEnum"=w547) -> ()  [unwired: 2 in, 2 out]
            n372 = property on="CV Step Interval [s]" class="DigNum (strict)"("DisabledEnum"=w547) -> ()  [unwired: 2 in, 2 out]
            n373 = local read "Y Mapping"() -> (w538:string[])
            n374 = global read "InstrumentSetup.vi" "MUX & Matrix Configurations"() -> (w523:T4)
            n375 = case shown="True" "Save CV defaults" {
              frame False {
              }
              frame True {
              }
            }
            n376 = Absolute Value(x="CV Final Voltage [V]") -> (abs(x)=w569:dbl)
            n377 = Absolute Value(x="CV Initial Voltage [V]") -> (abs(x)=w568:dbl)
            n378 = Replace Array Subset(array=w538, new element #1="Backplane" ("String"), index #1=0, new element #2="Bias Rail (GND)" ("String"), index #2=1, new element #3=w544, index #3=2, new element #4=w544, index #4=3) -> (w539:string[])
            n379 = Subtract(x=w569, y=w568) -> (x-y=w567:dbl)
            n380 = local write "Y Mapping"(w539) -> ()
            n381 = Unbundle By Name(w523) -> ("Matrix X Channels.Volt meter LO"=w521:i32, "Matrix X Channels.Volt meter HI"=w520:i32, "Matrix X Channels.Mux1 C1"=w527:i32, "Matrix X Channels.Mux1 C2"=w528:i32, "Matrix X Channels.Mux2 C1"=w525:i32, "Matrix X Channels.Mux2 C2"=w526:i32)
            n382 = Absolute Value(x=w567) -> (abs(x)=w566:dbl)
            n383 = Absolute Value(x="CV Step Size [V]") -> (abs(x)=w570:dbl)
            n384 = call "InstrumentSelection.vi"("Instrument type"=enum16{"Supply", "LCR", "Multimeter"}."Supply", "Instrument name IN"="CV Voltage Supply") -> ("error out"=w552:errorcluster, "Instrument name OUT"=w560:string, "Supply"=w558:refnum<class "SupplyControl.lvclass">)  [unwired: 5 in, 2 out]
            n385 = local read "X Mapping CB Standard"() -> (w524:string[])
            n386 = global read "QC_MeasurementSetup.vi" "CV Measurement Parameters"() -> (w575:T6)
            n387 = Quotient & Remainder(x=w566, y=w570) -> (floor(x/y)=w565:dbl)  [unwired: 1 out]
            n388 = Decrement(x=w521) -> (x-1=w530:i32)
            n389 = Decrement(x=w520) -> (x-1=w531:i32)
            n390 = Decrement(x=w527) -> (x-1=w532:i32)
            n391 = Decrement(x=w528) -> (x-1=w533:i32)
            n392 = Decrement(x=w525) -> (x-1=w534:i32)
            n393 = Decrement(x=w526) -> (x-1=w535:i32)
            n394 = call "InstrumentSelection.vi"("error in (no error)"=w552, "Instrument type"=enum16{"Supply", "LCR", "Multimeter"}."LCR", "Instrument name IN"="CV LCR Meter") -> ("Instrument name OUT"=w550:string, "LCR"=w551:refnum<class "LCRControl.lvclass">)  [unwired: 4 in, 3 out]
            n395 = Increment(x=w565) -> (x+1=w561:dbl)
            n396 = Replace Array Subset(array=w524, new element #1=w529, index #1=w530, new element #2=w529, index #2=w531, new element #3=w529, index #3=w532, new element #4=w529, index #4=w533, new element #5=w529, index #5=w534, new element #6=w529, index #6=w535) -> (w522:string[])
            n397 = local write "X Mapping"(w522) -> ()
            n398 = Bundle By Name(cluster=w575, "Supply"=w558, "LCR"=w551, "Initial Voltage [V]"="CV Initial Voltage [V]", "Final Voltage [V]"="CV Final Voltage [V]", "Step Size [V]"="CV Step Size [V]", "Step Interval [s]"="CV Step Interval [s]", "Number Of Steps"=w561, "RC Configuration"=w549, "Ramp down steps [V]"="CV Ramp down steps [V]", "Ramp down Interval [s]"="CV Ramp down Interval [s]", "Temperature Readout"="CV Temperature Readout", "Supply Name"=w560, "LCR Name"=w550, "V_depletion Limit [V]"="V_depletion Limit [V]") -> (w576:T6)
            n399 = global write "QC_MeasurementSetup.vi" "CV Measurement Parameters"(w576) -> ()
          }
          frame "Stability" {
            w580 = 11
            w588 = ""
            n400 = Select(t=0, s=w592, f=2) -> (s? t:f=w591:i32)
            n401 = property on="Maximum current fluctuation [%]" class="DigNum (strict)"("DisabledEnum"=w591) -> ()  [unwired: 2 in, 2 out]
            n402 = local read "X Mapping CB Standard"() -> (w581:string[])
            n403 = local read "Y Mapping"() -> (w583:string[])
            n404 = for {
              N: w580 -> [_]
              shift-right: [w601] -> w578
              shift-left: w581 -> [w602]
              i -> [w603]
              n405 = Increment(x=w603) -> (x+1=w599:i32)
              n406 = Format Into String(format string="Sensor %d", w599) -> (resulting string=w596:string)  [unwired: 2 in, 1 out]
              n407 = Less Or Equal?(x=w599, y=3) -> (x <= y?=w600:bool)
              n408 = Select(t=w596, s=w600, f="     ...     ") -> (s? t:f=w595:string)
              n409 = Replace Array Subset(array=w602, new element=w595, index=w603) -> (w601:string[])
            }
            n410 = Replace Array Subset(array=w583, new element #1="Amp meter HI" ("String"), index #1=0, new element #2="Bias Supply LO" ("String"), index #2=1, new element #3=w588, index #3=2, new element #4=w588, index #4=3) -> (w584:string[])
            n411 = local write "Y Mapping"(w584) -> ()
            n412 = Replace Array Subset(array=w578, new element="Amp meter LO", index=w580) -> (w577:string[])
            n413 = local write "X Mapping"(w577) -> ()
          }
          frame "Striptest" {
            w607 = "" ("Input Element")
            w627 = ""
            n414 = Select(t=0, s=w629, f=2) -> (s? t:f=w628:i32)
            n415 = property on="Fraction of good strips [%]" class="DigNum (strict)"("DisabledEnum"=w628) -> ()  [unwired: 2 in, 2 out]
            n416 = local read "Y Mapping"() -> (w621:string[])
            n417 = global read "InstrumentSetup.vi" "MUX & Matrix Configurations"() -> (w617:T4)
            n418 = Replace Array Subset(array=w621, new element #1="Probe Needle(s)" ("String"), index #1=0, new element #2="Common GND" ("String"), index #2=1, new element #3=w627, index #3=2, new element #4=w627, index #4=3) -> (w622:string[])
            n419 = local write "Y Mapping"(w622) -> ()
            n420 = Unbundle By Name(w617) -> ("Matrix X Channels.Bias Supply / SMU LO"=w616:i32, "Matrix X Channels.Bias Supply / SMU HI"=w615:i32, "Matrix X Channels.Volt meter LO"=w611:i32, "Matrix X Channels.Volt meter HI"=w610:i32)
            n421 = local read "X Mapping CB Standard"() -> (w618:string[])
            n422 = Decrement(x=w616) -> (x-1=w614:i32)
            n423 = Decrement(x=w615) -> (x-1=w612:i32)
            n424 = Decrement(x=w611) -> (x-1=w609:i32)
            n425 = Decrement(x=w610) -> (x-1=w608:i32)
            n426 = Replace Array Subset(array=w618, new element #1="SMU LO (GND)" ("Input Element"), index #1=w614, new element #2="SMU HI" ("Input Element"), index #2=w612, new element #3=w607, index #3=w609, new element #4=w607, index #4=w608) -> (w613:string[])
            n427 = local write "X Mapping"(w613) -> ()
          }
          frame "Cis" {
            w645 = "" ("Input Element")
            w662 = u16 1 items=["serial", "parallel"] ("RC Configuration")
            n428 = Select(t=0, s=w687, f=2) -> (s? t:f=w661:i32)
            n429 = property on="C_is Limit [pF/cm]" class="DigNum (strict)"("DisabledEnum"=w661) -> ()  [unwired: 2 in, 2 out]
            n430 = property on="Cis Ramp down Interval [s]" class="DigNum (strict)"("DisabledEnum"=w661) -> ()  [unwired: 2 in, 2 out]
            n431 = property on="Cis Initial Voltage [V]" class="DigNum (strict)"("DisabledEnum"=w661) -> ()  [unwired: 2 in, 2 out]
            n432 = property on="Cis Ramp down steps [V]" class="DigNum (strict)"("DisabledEnum"=w661) -> ()  [unwired: 2 in, 2 out]
            n433 = property on="Cis Final Voltage [V]" class="DigNum (strict)"("DisabledEnum"=w661) -> ()  [unwired: 2 in, 2 out]
            n434 = property on="Cis Step Size [V]" class="DigNum (strict)"("DisabledEnum"=w661) -> ()  [unwired: 2 in, 2 out]
            n435 = property on="Cis Step Interval [s]" class="DigNum (strict)"("DisabledEnum"=w661) -> ()  [unwired: 2 in, 2 out]
            n436 = local read "Y Mapping"() -> (w653:string[])
            n437 = global read "InstrumentSetup.vi" "MUX & Matrix Configurations"() -> (w639:T4)
            n438 = case shown="True" "Save Cis defaults" {
              frame False {
              }
              frame True {
              }
            }
            n439 = Absolute Value(x="Cis Final Voltage [V]") -> (abs(x)=w671:dbl)
            n440 = Absolute Value(x="Cis Initial Voltage [V]") -> (abs(x)=w670:dbl)
            n441 = Replace Array Subset(array=w653, new element #1="Backplane" ("String"), index #1=0, new element #2="Bias Rail (GND)" ("String"), index #2=1, new element #3="Neighbour Strips" ("String"), index #3=2, new element #4="Centre Strip" ("String"), index #4=3) -> (w654:string[])
            n442 = Subtract(x=w671, y=w670) -> (x-y=w669:dbl)
            n443 = local write "Y Mapping"(w654) -> ()
            n444 = Unbundle By Name(w639) -> ("Matrix X Channels.Volt meter LO"=w637:i32, "Matrix X Channels.Volt meter HI"=w636:i32, "Matrix X Channels.Mux1 C1"=w643:i32, "Matrix X Channels.Mux1 C2"=w644:i32, "Matrix X Channels.Mux2 C1"=w641:i32, "Matrix X Channels.Mux2 C2"=w642:i32)
            n445 = Absolute Value(x=w669) -> (abs(x)=w668:dbl)
            n446 = Absolute Value(x="Cis Step Size [V]") -> (abs(x)=w672:dbl)
            n447 = call "InstrumentSelection.vi"("Instrument type"=enum16{"Supply", "LCR", "Multimeter"}."Supply", "Instrument name IN"="Cis Voltage Supply") -> ("error out"=w683:errorcluster, "Instrument name OUT"=w679:string, "Supply"=w680:refnum<class "SupplyControl.lvclass">)  [unwired: 5 in, 2 out]
            n448 = local read "X Mapping CB Standard"() -> (w640:string[])
            n449 = global read "QC_MeasurementSetup.vi" "Cis Measurement Parameters"() -> (w685:T5)
            n450 = Quotient & Remainder(x=w668, y=w672) -> (floor(x/y)=w664:dbl)  [unwired: 1 out]
            n451 = Decrement(x=w637) -> (x-1=w646:i32)
            n452 = Decrement(x=w636) -> (x-1=w647:i32)
            n453 = Decrement(x=w643) -> (x-1=w648:i32)
            n454 = Decrement(x=w644) -> (x-1=w649:i32)
            n455 = Decrement(x=w641) -> (x-1=w650:i32)
            n456 = Decrement(x=w642) -> (x-1=w651:i32)
            n457 = call "InstrumentSelection.vi"("error in (no error)"=w683, "Instrument type"=enum16{"Supply", "LCR", "Multimeter"}."LCR", "Instrument name IN"="Cis LCR Meter") -> ("Instrument name OUT"=w678:string, "LCR"=w681:refnum<class "LCRControl.lvclass">)  [unwired: 4 in, 3 out]
            n458 = Increment(x=w664) -> (x+1=w663:dbl)
            n459 = Replace Array Subset(array=w640, new element #1=w645, index #1=w646, new element #2=w645, index #2=w647, new element #3=w645, index #3=w648, new element #4=w645, index #4=w649, new element #5=w645, index #5=w650, new element #6=w645, index #6=w651) -> (w638:string[])
            n460 = local write "X Mapping"(w638) -> ()
            n461 = Bundle By Name(cluster=w685, "Supply"=w680, "LCR"=w681, "Initial Voltage [V]"="Cis Initial Voltage [V]", "Final Voltage [V]"="Cis Final Voltage [V]", "Step Size [V]"="Cis Step Size [V]", "Step Interval [s]"="Cis Step Interval [s]", "Number Of Steps"=w663, "RC Configuration"=w662, "Ramp down steps [V]"="Cis Ramp down steps [V]", "Ramp down Interval [s]"="Cis Ramp down Interval [s]", "Temperature Readout"="Cis Temperature Readout", "Supply Name"=w679, "LCR Name"=w678, "C_is Limit [pF/cm]"="C_is Limit [pF/cm]") -> (w686:T5)
            n462 = global write "QC_MeasurementSetup.vi" "Cis Measurement Parameters"(w686) -> ()
          }
          frame "Ris" {
            w708 = "" ("Input Element")
            w751 = enum16{"Supply", "LCR", "Multimeter"}."Supply" ("Instrument type")
            n463 = Select(t=0, s=w727, f=2) -> (s? t:f=w726:i32)
            n464 = property on="Ris Initial Voltage [V]" class="DigNum (strict)"("DisabledEnum"=w726) -> ()  [unwired: 2 in, 2 out]
            n465 = property on="Ris Ramp down Interval [s]" class="DigNum (strict)"("DisabledEnum"=w726) -> ()  [unwired: 2 in, 2 out]
            n466 = property on="Ris Step Size [V]" class="DigNum (strict)"("DisabledEnum"=w726) -> ()  [unwired: 2 in, 2 out]
            n467 = property on="Ris Step Interval [s]" class="DigNum (strict)"("DisabledEnum"=w726) -> ()  [unwired: 2 in, 2 out]
            n468 = property on="Ris Ramp down steps [V]" class="DigNum (strict)"("DisabledEnum"=w726) -> ()  [unwired: 2 in, 2 out]
            n469 = property on="Ris Final Voltage [V]" class="DigNum (strict)"("DisabledEnum"=w726) -> ()  [unwired: 2 in, 2 out]
            n470 = property on="R_is Limit [MOhm]" class="DigNum (strict)"("DisabledEnum"=w726) -> ()  [unwired: 2 in, 2 out]
            n471 = local read "Y Mapping"() -> (w717:string[])
            n472 = global read "InstrumentSetup.vi" "MUX & Matrix Configurations"() -> (w698:T4)
            n473 = case shown="True" "Save Ris defaults" {
              frame False {
              }
              frame True {
              }
            }
            n474 = Absolute Value(x="Ris Final Voltage [V]") -> (abs(x)=w741:dbl)
            n475 = Absolute Value(x="Ris Initial Voltage [V]") -> (abs(x)=w740:dbl)
            n476 = Subtract(x=w741, y=w740) -> (x-y=w739:dbl)
            n477 = call "InstrumentSelection.vi"("Instrument type"=w751, "Instrument name IN"="Ris Bias Supply") -> ("error out"=w753:errorcluster, "Instrument name OUT"=w747:string, "Supply"=w750:refnum<class "SupplyControl.lvclass">)  [unwired: 5 in, 2 out]
            n478 = Replace Array Subset(array=w717, new element #1="Centre Strip" ("String"), index #1=0, new element #2="High Strip" ("String"), index #2=1, new element #3="Ground Strip" ("String"), index #3=2, new element #4="", index #4=3) -> (w718:string[])
            n479 = Unbundle By Name(w698) -> ("Matrix X Channels.Bias Supply / SMU LO"=w710:i32, "Matrix X Channels.Bias Supply / SMU HI"=w711:i32, "Matrix X Channels.CV Box LO"=w694:i32, "Matrix X Channels.CV Box HI"=w695:i32, "Matrix X Channels.CV Box LO IN"=w696:i32, "Matrix X Channels.CV Box HI IN"=w693:i32, "Matrix X Channels.Mux1 C1"=w702:i32, "Matrix X Channels.Mux1 C2"=w703:i32, "Matrix X Channels.Mux2 C1"=w700:i32, "Matrix X Channels.Mux2 C2"=w701:i32)
            n480 = Absolute Value(x="Ris Step Size [V]") -> (abs(x)=w735:dbl)
            n481 = Absolute Value(x=w739) -> (abs(x)=w736:dbl)
            n482 = local read "X Mapping CB Standard"() -> (w699:string[])
            n483 = global read "QC_MeasurementSetup.vi" "Ris Measurement Parameters"() -> (w759:T7)
            n484 = local write "Y Mapping"(w718) -> ()
            n485 = Quotient & Remainder(x=w736, y=w735) -> (floor(x/y)=w733:dbl)  [unwired: 1 out]
            n486 = Decrement(x=w710) -> (x-1=w712:i32)
            n487 = Decrement(x=w711) -> (x-1=w713:i32)
            n488 = Decrement(x=w694) -> (x-1=w709:i32)
            n489 = Decrement(x=w695) -> (x-1=w690:i32)
            n490 = Decrement(x=w696) -> (x-1=w691:i32)
            n491 = Decrement(x=w693) -> (x-1=w692:i32)
            n492 = Decrement(x=w702) -> (x-1=w704:i32)
            n493 = Decrement(x=w703) -> (x-1=w705:i32)
            n494 = Decrement(x=w700) -> (x-1=w706:i32)
            n495 = Decrement(x=w701) -> (x-1=w707:i32)
            n496 = call "InstrumentSelection.vi"("error in (no error)"=w753, "Instrument type"=w751, "Instrument name IN"="Ris SMU") -> ("error out"=w752:errorcluster, "Instrument name OUT"=w746:string, "Supply"=w749:refnum<class "SupplyControl.lvclass">)  [unwired: 4 in, 2 out]
            n497 = call "InstrumentSelection.vi"("error in (no error)"=w752, "Instrument type"=enum16{"Supply", "LCR", "Multimeter"}."Multimeter", "Instrument name IN"="Ris Voltmeter") -> ("Instrument name OUT"=w745:string, "Multimeter"=w748:refnum<class "MultimeterControl.lvclass">)  [unwired: 4 in, 3 out]
            n498 = Increment(x=w733) -> (x+1=w732:dbl)
            n499 = Bundle By Name(cluster=w759, "Bias Supply"=w750, "SMU"=w749, "Multimeter"=w748, "Initial Voltage [V]"="Ris Initial Voltage [V]", "Final Voltage [V]"="Ris Final Voltage [V]", "Step Size [V]"="Ris Step Size [V]", "Step Interval [s]"="Ris Step Interval [s]", "Number Of Steps"=w732, "Ramp down steps [V]"="Ris Ramp down steps [V]", "Ramp down Interval [s]"="Ris Ramp down Interval [s]", "Temperature Readout"="Ris Temperature Readout", "Supply Name"=w747, "SMU Name"=w746, "Voltmeter Name"=w745, "R_is Limit [MOhm]"="R_is Limit [MOhm]") -> (w758:T7)
            n500 = Replace Array Subset(array=w699, new element #1="SMU LO (GND)" ("Input Element"), index #1=w712, new element #2="SMU HI" ("Input Element"), index #2=w713, new element #3=w708, index #3=w709, new element #4=w708, index #4=w690, new element #5=w708, index #5=w691, new element #6=w708, index #6=w692, new element #7=w708, index #7=w704, new element #8=w708, index #8=w705, new element #9=w708, index #9=w706, new element #10=w708, index #10=w707) -> (w697:string[])
            n501 = global write "QC_MeasurementSetup.vi" "Ris Measurement Parameters"(w758) -> ()
            n502 = local write "X Mapping"(w697) -> ()
          }
          frame "PTP" {
            w769 = ""
            n503 = local read "X Mapping CB Standard"() -> (w761:string[])
            n504 = local read "Y Mapping"() -> (w767:string[])
            n505 = local write "X Mapping"(w761) -> ()
            n506 = Replace Array Subset(array=w767, new element #1="MUX" ("String"), index #1=0, new element #2="Common GND" ("String"), index #2=1, new element #3=w769, index #3=2, new element #4=w769, index #4=3) -> (w764:string[])
            n507 = local write "Y Mapping"(w764) -> ()
          }
        }
        n508 = local write "Change Preset Parameters"(w164) -> ()
      }
      n509 = local write "configured?"(w127) -> ()
    }
  }
